vi "MainGUI.vi"() -> ()   [LabVIEW 2018]
uses:
  General/Controls/ScanType.ctl
  General/Controls/Vibratome Parameters.ctl
  General/type defines/vibratome.ctl
  General/Controls/Imaging Parameters.ctl
  General/Controls/Scan Direction.ctl
  General/type defines/Alazar parameters.ctl
  Hardware Mfg/AlazarTech SDK/Controls/General Trigger Settings.ctl
  Hardware Mfg/AlazarTech SDK/Controls/Trigger Engine Controls.ctl
  Hardware Mfg/AlazarTech SDK/Controls/Alazar Device ID.ctl
  Hardware Mfg/AlazarTech SDK/Controls/Channel Input Controls.ctl
  Hardware Mfg/AlazarTech SDK/Controls/Alazar Acquisition Settings.ctl
  Hardware Mfg/AlazarTech SDK/Controls/Clock Controls.ctl
  General/type defines/Galvo HW Parameters.ctl
  General/Controls/Optical Parameters.ctl
  General/Controls/Translation Stage Parameters.ctl
  Hardware Mfg/Thorlabs Translation Stages/Controls/Translation Stage Cluster.ctl
  General/Controls/Translation Stage Types.ctl
  General/type defines/Manual Controls.ctl
  General/type defines/FFT parameters.ctl
  General/type defines/FFT mode.ctl
  General/type defines/GPU FFT outputs.ctl
  General/type defines/Vibratome Param.ctl
  General/type defines/attenuator.ctl
  C:/Project/SerialSectionOCT/SerialSectOCT/Labview Software/Thorlabs.MotionControl.Controls.dll
  Thorlabs.MotionControl.Controls.dll
  General/Controls/Queue Manager Actions.ctl
  General/Controls/MessagePacket.ctl
  General/Controls/QueueNames.ctl
  General/Controls/FGV Actions.ctl
  General/Controls/Save Bline to Mem Control.ctl
  General/Tile naming actions.ctl
  General/type defines/Pause action.ctl
  Hardware Mfg/Thorlabs Cage Rotation/refnum control.ctl
  General/Controls/Set Get Controls.ctl
  Hardware Mfg/Thorlabs Translation Stages/Controls/Motion Translation Module Control2.ctl
  General/Controls/file variable action.ctl
  Hardware Mfg/Main Scan Processor Status.vi
  Hardware Mfg/Axsun Laser/Axsun action.ctl
panel:
  in  "Status":string
  in  "Quit":bool
  in  "Acquire":bool
  in  "Control Panel":T1(tab)
  in  "Optical Parameters":T2={"Obj. Focal Length [mm]"=45.0, "Scan Lens EFL[mm]"=59.5, "Tube Lens EFL[mm]"=205.0, "Galvo V Range (+/-)"=10.0, "Galvo Max Half Angle [Deg]"=19.0, "Max Galvo Range[%]"=0.0}
  in  "Galvo HW Parameters":T3={"Analog Out Channel"="GalvoCtrl/ao0,GalvoCtrl/ao1", "Min Voltage"=-10.0, "Max Voltage"=10.0, "Pixel Clock Source"="/GalvoCtrl/PFI0", "Sample Rate"=1000.0, "Line Clock Out Ch(s)"="GalvoCtrl/port0/line0", "2P ready check"="Dev1/port0/line0:7"}
  in  "Imaging Parameter":T4={"Raster Scan Direction"=enum."Uni Directional", "Pixel Dwell Time [Clock Cycles]"=1, "Flyback Time [Clock Cycles]"=150, "XY Center [um]"={"X"=550.0, "Y"=450.0}, "Pixel Step Size [um] X"=3.0, "XY Image Size"=enum."2048 x 2048", "Custom"=TRUE, "Custom Size"={"X"=1050, "Y"=30}, "Line Averages"=1, "Pixel Step Size [um] Y"=0.0} {"Pixel Step Size [um] Y" min=0.0 max=100.0 step=0.01; "Line Averages" min=1 max=30 step=1; "Flyback Time [Clock Cycles]" max=1000 step=1; "Pixel Step Size [um] X" min=0.0 max=100.0 step=0.01; "Custom Size"."Y" min=2 max=10000 step=1; "Custom Size"."X" min=1 max=30 step=1; "XY Center [um]"."Y" min=1.0 max=30.0 step=1.0; "XY Center [um]"."X" min=1.0 max=30.0 step=1.0; "Pixel Dwell Time [Clock Cycles]" max=10 step=1}
  in  "Scan Type":T6
  in  "Alazar parameters":T7={"Trigger Settings"={"General Trigger Settings"={"Trigger Operation"=0, "Coupling ID"=2, "Range ID"=2, "Delay"=0, "Timeout Ticks"=0, "Mode"=1, "Parameter"=1}, "Trigger Engine 1"={"Trigger Engine"=0, "Source"=2, "Slope"=1, "Level"=140}, "Trigger Engine 2"={"Trigger Engine"=1, "Source"=2, "Slope"=1, "Level"=2048}}, "Device ID"={"System ID"=1, "Board ID"=1}, "Ch A Input Control"={"Channel"=1, "Coupling"=2, "Range"=7, "Impedance"=2}, "Ch B Input Control"={"Channel"=2, "Coupling"=2, "Range"=7, "Impedance"=2}, "Acq Settings"={"Record Length"=1440, "Offset"=0, "Records Per Buffer"=1100, "Records Count (Records/Acq)"=2147483647, "Window Type"=1, "Footer"=0, "Samples per record"=2048, "Output Format"=11}, "Capture Clock"={"Sample Rate"=100, "Decimation"=0, "Source"=2, "Edge"=0}} {"Capture Clock"."Edge" items=["Rising", "Falling"]; "Capture Clock"."Source" items=["Internal"=1, "Fast External"=2, "Medium External"=3, "Slow External"=4, "External AC"=5, "External DC"=6, "External 10MHz"=7]; "Acq Settings"."Output Format" items=["Float Log"=11, "Float Amp"=10, "U16_LOG"=1, "U16_AMP2"=257, "Real"=3, "Imag"=4]; "Acq Settings"."Footer" items=["FOOTER_NONE", "FOOTER_NPT"]; "Acq Settings"."Window Type" items=["DSP_WINDOW_NONE", "DSP_WINDOW_HANNING", "DSP_WINDOW_HAMMING", "DSP_WINDOW_BLACKMAN", "DSP_WINDOW_BLACKMAN_HARRIS", "DSP_WINDOW_BARTLETT"]; "Ch B Input Control"."Channel" items=["A"=1, "B"=2, "C"=4, "D"=8]; "Ch B Input Control"."Coupling" items=["AC"=1, "DC"=2]; "Ch B Input Control"."Range" items=["20 mV"=1, "40 mV"=2, "50 mV"=3, "80 mV"=4, "100 mV"=5, "200 mV"=6, "400 mV"=7, "500 mV"=8, "800 mV"=9, "1 V"=10, "1.25 V"=33, "2 V"=11, "4 V"=12, "5 V"=13, "8 V"=14, "10 V"=15, "20 V"=16]; "Ch B Input Control"."Impedance" items=["1 MOhm"=1, "50 Ohm"=2, ""=0]; "Ch A Input Control"."Channel" items=["A"=1, "B"=2, "C"=4, "D"=8]; "Ch A Input Control"."Coupling" items=["AC"=1, "DC"=2]; "Ch A Input Control"."Range" items=["20 mV"=1, "40 mV"=2, "50 mV"=3, "80 mV"=4, "100 mV"=5, "200 mV"=6, "400 mV"=7, "500 mV"=8, "800 mV"=9, "1 V"=10, "1.25 V"=33, "2 V"=11, "4 V"=12, "5 V"=13, "8 V"=14, "10 V"=15, "20 V"=16]; "Ch A Input Control"."Impedance" items=["1 MOhm"=1, "50 Ohm"=2, ""=0]; "Trigger Settings"."General Trigger Settings"."Trigger Operation" items=["J", "K", "J OR K", "J AND K", "J XOR K", "J AND NOT K", "NOT J AND K"]; "Trigger Settings"."General Trigger Settings"."Coupling ID" items=["AC"=1, "DC"=2]; "Trigger Settings"."General Trigger Settings"."Range ID" items=["5 V", "1 V", "TTL"]; "Trigger Settings"."Trigger Engine 1"."Trigger Engine" items=["J", "K"]; "Trigger Settings"."Trigger Engine 1"."Source" items=["A", "B", "External", "Disable", "C", "D"]; "Trigger Settings"."Trigger Engine 1"."Slope" items=["Positive"=1, "Negative"=2]; "Trigger Settings"."Trigger Engine 2"."Trigger Engine" items=["J", "K"]; "Trigger Settings"."Trigger Engine 2"."Source" items=["A", "B", "External", "Disable", "C", "D"]; "Trigger Settings"."Trigger Engine 2"."Slope" items=["Positive"=1, "Negative"=2]}
  in  "Z stage settings":T14={"first cut height(mm)"=45.85, "slice thickness[um]"=[], "#repetitions"=111, "image thickness(um)"=[], "#cycles per repetition"=0, "First image height(mm)"=2.1, "Block?"=[], "Z0"=0.0, "fixed Z0?"=FALSE}
  in  "Vibratome":T15={"Pre Cut Dwell [s]"=0.0, "Blade Frequency [RPM]"=0, "Slice Speed [mm/s]"=0.0, "Post Cut Dwell [s]"=0.0, "Ramp Time [s]"=10.0, "Start X [mm]"=0.0, "Start Y [mm]"=0.0, "Slice Length [mm]"=0.0, "Slice Axis"=enum."X Axis", "Controller VISA Ref"="COM4", "Blade Frequency [Hz]"=0, "Analog Out Channel"="GalvoCtrl/ao0,GalvoCtrl/ao1", "Pixel Clock Source"="/GalvoCtrl/PFI0", "Vib version"=enum."Vibratome1"} {"Start X [mm]" min=10.0; "Slice Speed [mm/s]" format="%.2f"}
  in  "Mosaic Paramter":T17={"X Axis"={"Start [mm]"=56.0, "FOV[mm]"=3.0, "End [mm]"=70.8}, "Y Axis"={"Start [mm]"=102.5, "FOV[mm]"=3.0, "End [mm]"=117.2}, "Scan Pattern"=enum."Uni-directional", "Overlap Options"={"Overlap Type"=enum."X and Y", "Percent Overlap"=10, "Justify"=enum."Start"}}
  in  "Attenuator":T18
  in  "Manual Controls":T19={"Data Path"=path "C:/Users/BOAS-USER/Documents/Data/0922", "Save parameters"={"start pixel"=45, "#pixels to save"=100}, "Acquisition mode"=enum."Alazar FFT", "PSOCT Channel"=1, "Save data?"=FALSE, "AIP rotation angle"=0.0, "Pause acquisition?"=FALSE, "Outgoing Mail Server (SMTP)"="smtp.gmail.com", "Email"="nauge7811@gmail.com", "Password"="csb19960128", "Carrier 1"=enum."Sprint", "phone number 1"="8578002084", "Subject"="", "Message"="Brain slice: stop watching Netflix, come and pick me up!", "Carrier 2"=enum."Sprint", "phone number 2"="", "Check boundary?"=FALSE, "Threshold"=0.0, "Outputs for GPU FFT"=enum."Amp + Phase diff"} {"PSOCT Channel" items=["A"=1, "B"=2, "A + B"=3, "C"=4, "A + C"=5, "A + B"=6, "D"=8, "A + D"=9, "B + D"=10, "C + D"=12, "A + B + C + D"=15]}
  in  "Table Stages":T23={"X Stage"={"Position"=0.0, "Is.Enabled?"=FALSE, "Is.Connected?"=FALSE, "Device SN"="45876425", "AccelerationMaximum"=20.0, "VelocityMaximum"=20.0, "Acceleration"=10.0, "Velocity"=10.0, "waitTimeout (ms)"=1000000, "Model"=enum."Thorlabs LTS", "Is.Homed?"=FALSE, "MOVE"=FALSE}, "Y Stage"={"Position"=0.0, "Is.Enabled?"=FALSE, "Is.Connected?"=FALSE, "Device SN"="45995820", "AccelerationMaximum"=20.0, "VelocityMaximum"=20.0, "Acceleration"=10.0, "Velocity"=10.0, "waitTimeout (ms)"=10000000, "Model"=enum."Thorlabs LTS", "Is.Homed?"=FALSE, "MOVE"=FALSE}, "Z Stage"={"Position"=0.0, "Is.Enabled?"=FALSE, "Is.Connected?"=FALSE, "Device SN"="49103464", "AccelerationMaximum"=8.0, "VelocityMaximum"=3.0, "Acceleration"=4.0, "Velocity"=2.0, "waitTimeout (ms)"=1000000, "Model"=enum."Thorlabs MLJ", "Is.Homed?"=FALSE, "MOVE"=FALSE}, "Attenuator"={"Position"=0.0, "Is.Enabled?"=FALSE, "Is.Connected?"=FALSE, "Device SN"="45876539", "AccelerationMaximum"=0.0, "VelocityMaximum"=0.0, "Acceleration"=0.0, "Velocity"=0.0, "waitTimeout (ms)"=0, "Model"=enum."None", "Is.Homed?"=FALSE, "MOVE"=FALSE}}
  in  "Attenuator":refnum<k24>(container)
  out "XY Graph out":cluster{"X":dbl, "Y":dbl}[](graph)
  out "AIP":T26(plugin-control) caption="Image"
  out "wanring":string="test"
  out "attenuator angle":dbl
  in  "attenuator power(mW)":dbl=300.0 format="%#_13g"
  out "requested 2P power out":dbl
  out "attenuator angle out":dbl
  out "tile average intensity":dbl
  in  "Init Tables":bool
  out "Current Position out":cluster{"X":dbl, "Y":dbl, "Z":dbl}
  out "slice plane out":dbl
  out "image plane out":dbl
  # "Image Settings"
  # "Optical Settings"
  # "X"
  # "X"
  # "(mW)"
  # "Vibratome Settings"
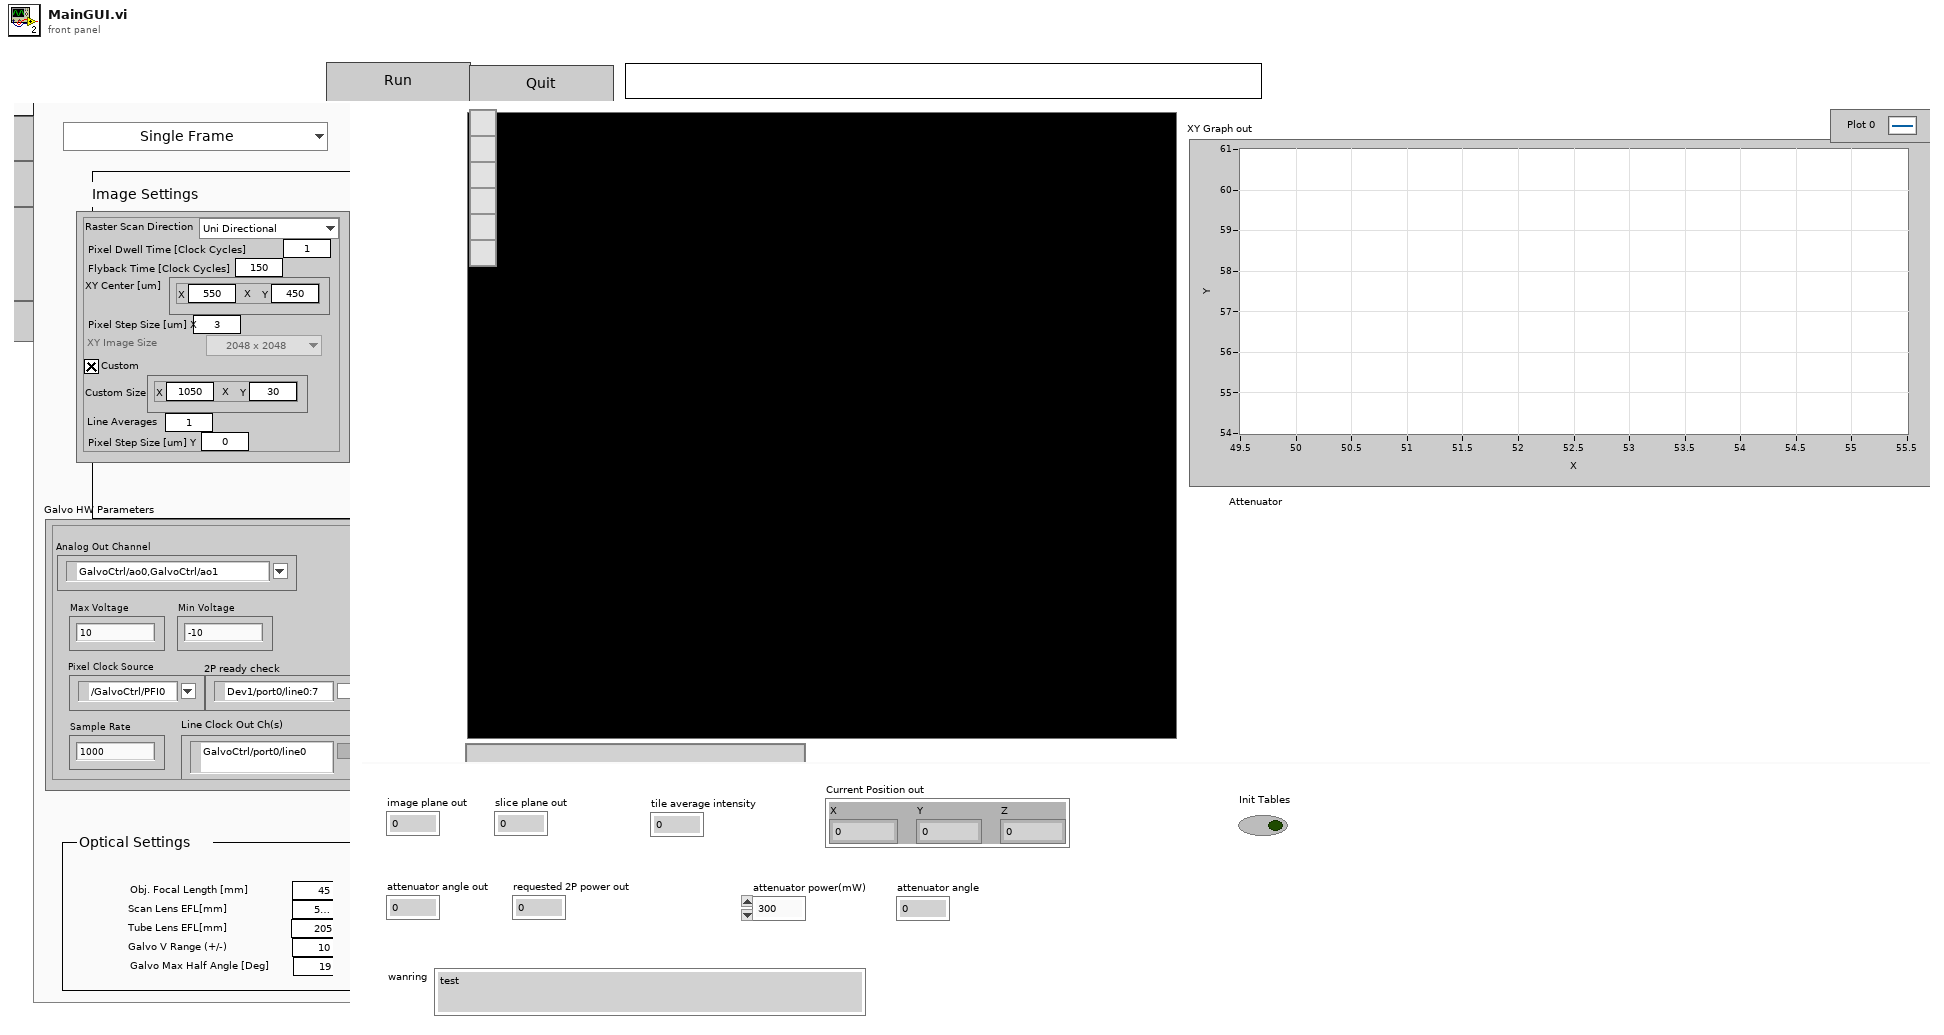
[diagram p1: front panel]
types:
  T1 = enum32{"Galvo", "Alazar", "Config", "Manual Contorls", "Table"}
  T2 = typedef "Optical Parameters.ctl" = cluster{"Obj. Focal Length [mm]":dbl, "Scan Lens EFL[mm]":dbl, "Tube Lens EFL[mm]":dbl, "Galvo V Range (+/-)":dbl, "Galvo Max Half Angle [Deg]":dbl, "Max Galvo Range[%]":dbl}
  T3 = typedef "Galvo HW Parameters.ctl" = cluster{"Analog Out Channel":tag, "Min Voltage":dbl, "Max Voltage":dbl, "Pixel Clock Source":tag, "Sample Rate":dbl, "Line Clock Out Ch(s)":tag, "2P ready check":tag}
  T4 = typedef "Imaging Parameters.ctl" = cluster{"Raster Scan Direction":T5, "Pixel Dwell Time [Clock Cycles]":u16, "Flyback Time [Clock Cycles]":u16, "XY Center [um]":cluster{"X":dbl, "Y":dbl}, "Pixel Step Size [um] X":dbl, "XY Image Size":enum16{"32 x 32", "64 x 64", "128 x 128", "256 x 256", "512 x 512", "1024 x 1024", "2048 x 2048"}, "Custom":bool, "Custom Size":cluster{"X":u16, "Y":u16}, "Line Averages":u16, "Pixel Step Size [um] Y":dbl}
  T5 = typedef "Scan Direction.ctl" = enum16{"Uni Directional", "Bi Directional", "None"}
  T6 = typedef "ScanType.ctl" = enum16{"Single Frame", "Continuous Frame", "ROI Line", "Vibratome", "Mosaic", "Mosaic + Slice"}
  T7 = typedef "Alazar parameters.ctl" = cluster{"Trigger Settings":cluster{"General Trigger Settings":T8, "Trigger Engine 1":T9, "Trigger Engine 2":T9}, "Device ID":T10, "Ch A Input Control":T11, "Ch B Input Control":T11, "Acq Settings":T12, "Capture Clock":T13}
  T8 = typedef "General Trigger Settings.ctl" = cluster{"Trigger Operation":u32, "Coupling ID":u32, "Range ID":u32, "Delay":u32, "Timeout Ticks":u32, "Mode":u32, "Parameter":u32}
  T9 = typedef "Trigger Engine Controls.ctl" = cluster{"Trigger Engine":u32, "Source":u32, "Slope":u32, "Level":u32}
  T10 = typedef "Alazar Device ID.ctl" = cluster{"System ID":u32, "Board ID":u32}
  T11 = typedef "Channel Input Controls.ctl" = cluster{"Channel":u8, "Coupling":u32, "Range":u32, "Impedance":u32}
  T12 = typedef "Alazar Acquisition Settings.ctl" = cluster{"Record Length":u32, "Offset":u32, "Records Per Buffer":u32, "Records Count (Records/Acq)":u32, "Window Type":u32, "Footer":u32, "Samples per record":u32, "Output Format":u32}
  T13 = typedef "Clock Controls.ctl" = cluster{"Sample Rate":u32, "Decimation":u32, "Source":u32, "Edge":u32}
  T14 = typedef "Vibratome Param.ctl" = cluster{"first cut height(mm)":dbl, "slice thickness[um]":dbl[], "#repetitions":u16, "image thickness(um)":dbl[], "#cycles per repetition":u16, "First image height(mm)":dbl, "Block?":bool[], "Z0":dbl, "fixed Z0?":bool}
  T15 = typedef "Vibratome Parameters.ctl" = cluster{"Pre Cut Dwell [s]":dbl, "Blade Frequency [RPM]":u16, "Slice Speed [mm/s]":dbl, "Post Cut Dwell [s]":dbl, "Ramp Time [s]":dbl, "Start X [mm]":dbl, "Start Y [mm]":dbl, "Slice Length [mm]":dbl, "Slice Axis":enum16{"X Axis", "Y Axis", "Z Axis"}, "Controller VISA Ref":refnum<visa-resource-name>, "Blade Frequency [Hz]":u16, "Analog Out Channel":tag, "Pixel Clock Source":tag, "Vib version":T16}
  T16 = typedef "vibratome.ctl" = enum16{"Vibratome1", "Vibratome3"}
  T17 = cluster{"X Axis":cluster{"Start [mm]":dbl, "FOV[mm]":dbl, "End [mm]":dbl}, "Y Axis":cluster{"Start [mm]":dbl, "FOV[mm]":dbl, "End [mm]":dbl}, "Scan Pattern":enum16{"Uni-directional", "Bi-Directional", "Spiral Out", "Spiral In"}, "Overlap Options":cluster{"Overlap Type":enum16{"No Overlap", "X Only", "Y Only", "X and Y"}, "Percent Overlap":u8, "Justify":enum16{"Start", "Center", "End"}}}
  T18 = typedef "attenuator.ctl" = cluster{"Power after Objective (recalibrate every 6 month)":dbl[]}
  T19 = typedef "Manual Controls.ctl" = cluster{"Data Path":path, "Save parameters":T20, "Acquisition mode":T21, "PSOCT Channel":u32, "Save data?":bool, "AIP rotation angle":dbl, "Pause acquisition?":bool, "Outgoing Mail Server (SMTP)":string, "Email":string, "Password":string, "Carrier 1":enum16{"T-Mobile", "AT&T", "Verizon", "Sprint"}, "phone number 1":string, "Subject":string, "Message":string, "Carrier 2":enum16{"T-Mobile", "AT&T", "Verizon", "Sprint"}, "phone number 2":string, "Check boundary?":bool, "Threshold":sgl, "Outputs for GPU FFT":T22}
  T20 = typedef "FFT parameters.ctl" = cluster{"start pixel":i32, "#pixels to save":i32}
  T21 = typedef "FFT mode.ctl" = enum16{"ThorOCT B line", "ThorOCT Spectral", "ThorOCT FFT", "Alazar B line", "Alazar FFT", "GPU FFT", "Alazar Spectral", "Simulation", "auto adjust focus", "Save all"}
  T22 = typedef "GPU FFT outputs.ctl" = enum16{"Amp + Phase diff", "Amp + Phase", "Amp only"}
  T23 = typedef "Translation Stage Parameters.ctl" = cluster{"X Stage":T24, "Y Stage":T24, "Z Stage":T24, "Attenuator":T24}
  T24 = typedef "Translation Stage Cluster.ctl" = cluster{"Position":dbl, "Is.Enabled?":bool, "Is.Connected?":bool, "Device SN":string, "AccelerationMaximum":dbl, "VelocityMaximum":dbl, "Acceleration":dbl, "Velocity":dbl, "waitTimeout (ms)":i32, "Model":T25, "Is.Homed?":bool, "MOVE":bool}
  T25 = typedef "Translation Stage Types.ctl" = enum16{"None", "Thorlabs LTS", "Thorlabs MLJ"}
  T26 = typedef "IMAQ Image.ctl" = refnum<image>
  T27 = enum16{"Create file", "Write config", "Write log", "Close file"}
  T28 = typedef "Queue Manager Actions.ctl" = enum16{"Init", "Enqueue", "Enqueue All", "Preview Queue", "Dequeue", "Get Status", "Flush Queue", "Flush All Queues", "Release All Queues", "Release Queue", "Enqueue at Opposite End"}
  T29 = typedef "QueueNames.ctl" = enum16{"Main GUI", "Main Scan Processor", "Main Processing", "Main Saving", "Main Display", "Main Table Stage GUI", "Main Table Stage Proc.", "Scan Engine", "Vibratome GUI", "Vibratome Processor", "Slice Engine"}
  T30 = typedef "MessagePacket.ctl" = cluster{"Message":string, "Parameter":variant}
  T31 = typedef "FGV Actions.ctl" = enum16{"Init", "Set", "Get", "Clear"}
  T32 = typedef "Image Type" = u32
  T33 = typedef "System Parameters.ctl" = cluster{"Optical Parameters":T2, "Vibratome":T15, "Table Stages":T23, "Imaging Parameter":T4, "Galvo HW Parameters":cluster{"Analog Out Channel":tag, "Min Voltage":dbl, "Max Voltage":dbl, "Pixel Clock Source":tag, "Sample Rate":dbl, "Line Clock Out Ch":tag, "2P ready check":tag}, "Alazar parameters":T7, "Mosaic Paramter":cluster{"X Axis":cluster{"Start [mm]":dbl, "Steps [pts]":dbl, "End [mm]":dbl}, "Y Axis":cluster{"Start [mm]":dbl, "Steps [pts]":dbl, "End [mm]":dbl}, "Scan Pattern":enum16{"Uni-directional", "Bi-Directional", "Spiral Out", "Spiral In"}, "Overlap Options":cluster{"Overlap Type":enum16{"No Overlap", "X Only", "Y Only", "X and Y"}, "Percent Overlap":u8, "Justify":enum16{"Start", "Center", "End"}}}, "Manual Controls":T19, "Z stage setting":T14, "Attenuator":T18}
  T34 = typedef "file variable action.ctl" = enum16{"File name", "X stage", "Y stage", "Slice plane", "Image plane", "time", "output", "Init", "Memory Usage", "Disk full Space", "Disk free space"}
  T35 = typedef "Pause action.ctl" = enum16{"Init", "get", "set"}
  T36 = typedef "Tile naming actions.ctl" = enum16{"Export", "Increment", "Total tile num", "Init"}
  T37 = typedef "Axsun action.ctl" = enum16{"GetSystemStatus", "Clock delay", "GetLaserOnTime", "GetWaveLengthAtSweptTrigger", "Source current ON", "GetSerialNum", "GetControlVersion", "Laser ON", "Laser OFF", "Source current OFF", "Get laser handle", "Start Network Control Interface", "stop", "Create handle"}
  T38 = typedef "Save Bline to Mem Control.ctl" = enum16{"Output data", "Save(ThorOCT)", "Save(PSOCT)", "FFT and Save", "Uninit", "PSOCT Spectral buffer Set", "PSOCT Spatial buffer Set", "PSOCT Spectral buffer Init", "PSOCT Spatial buffer Init", "ThorOCT Spectral buffer Init", "ThorOCT Spatial buffer Init", "ThorOCT Spectral buffer Set", "ThorOCT Spatial buffer Set", "ThorOCT Spectral Save", "Alazar Spectral Save", "PSOCT save all", "Average"}
  T39 = typedef "refnum control.ctl" = enum16{"Get", "Init"}
  T40 = typedef "Motion Translation Module Control2.ctl" = enum16{"Init", "Home", "Status", "Velocity/Accel", "Position", "Jog", "Stop", "Uninit", "Enable", "Disable"}
  T41 = typedef "Set Get Controls.ctl" = enum16{"Set", "Get"}
  T42 = cluster{"Analog Out Channel":tag, "Min Voltage":dbl, "Max Voltage":dbl, "Pixel Clock Source":tag, "Sample Rate":dbl, "Line Clock Out Ch":tag, "2P ready check":tag}
  T43 = cluster{"X Axis":cluster{"Start [mm]":dbl, "Steps [pts]":dbl, "End [mm]":dbl}, "Y Axis":cluster{"Start [mm]":dbl, "Steps [pts]":dbl, "End [mm]":dbl}, "Scan Pattern":enum16{"Uni-directional", "Bi-Directional", "Spiral Out", "Spiral In"}, "Overlap Options":cluster{"Overlap Type":enum16{"No Overlap", "X Only", "Y Only", "X and Y"}, "Percent Overlap":u8, "Justify":enum16{"Start", "Center", "End"}}}
  T44 = enum16{"32 x 32", "64 x 64", "128 x 128", "256 x 256", "512 x 512", "1024 x 1024", "2048 x 2048"}
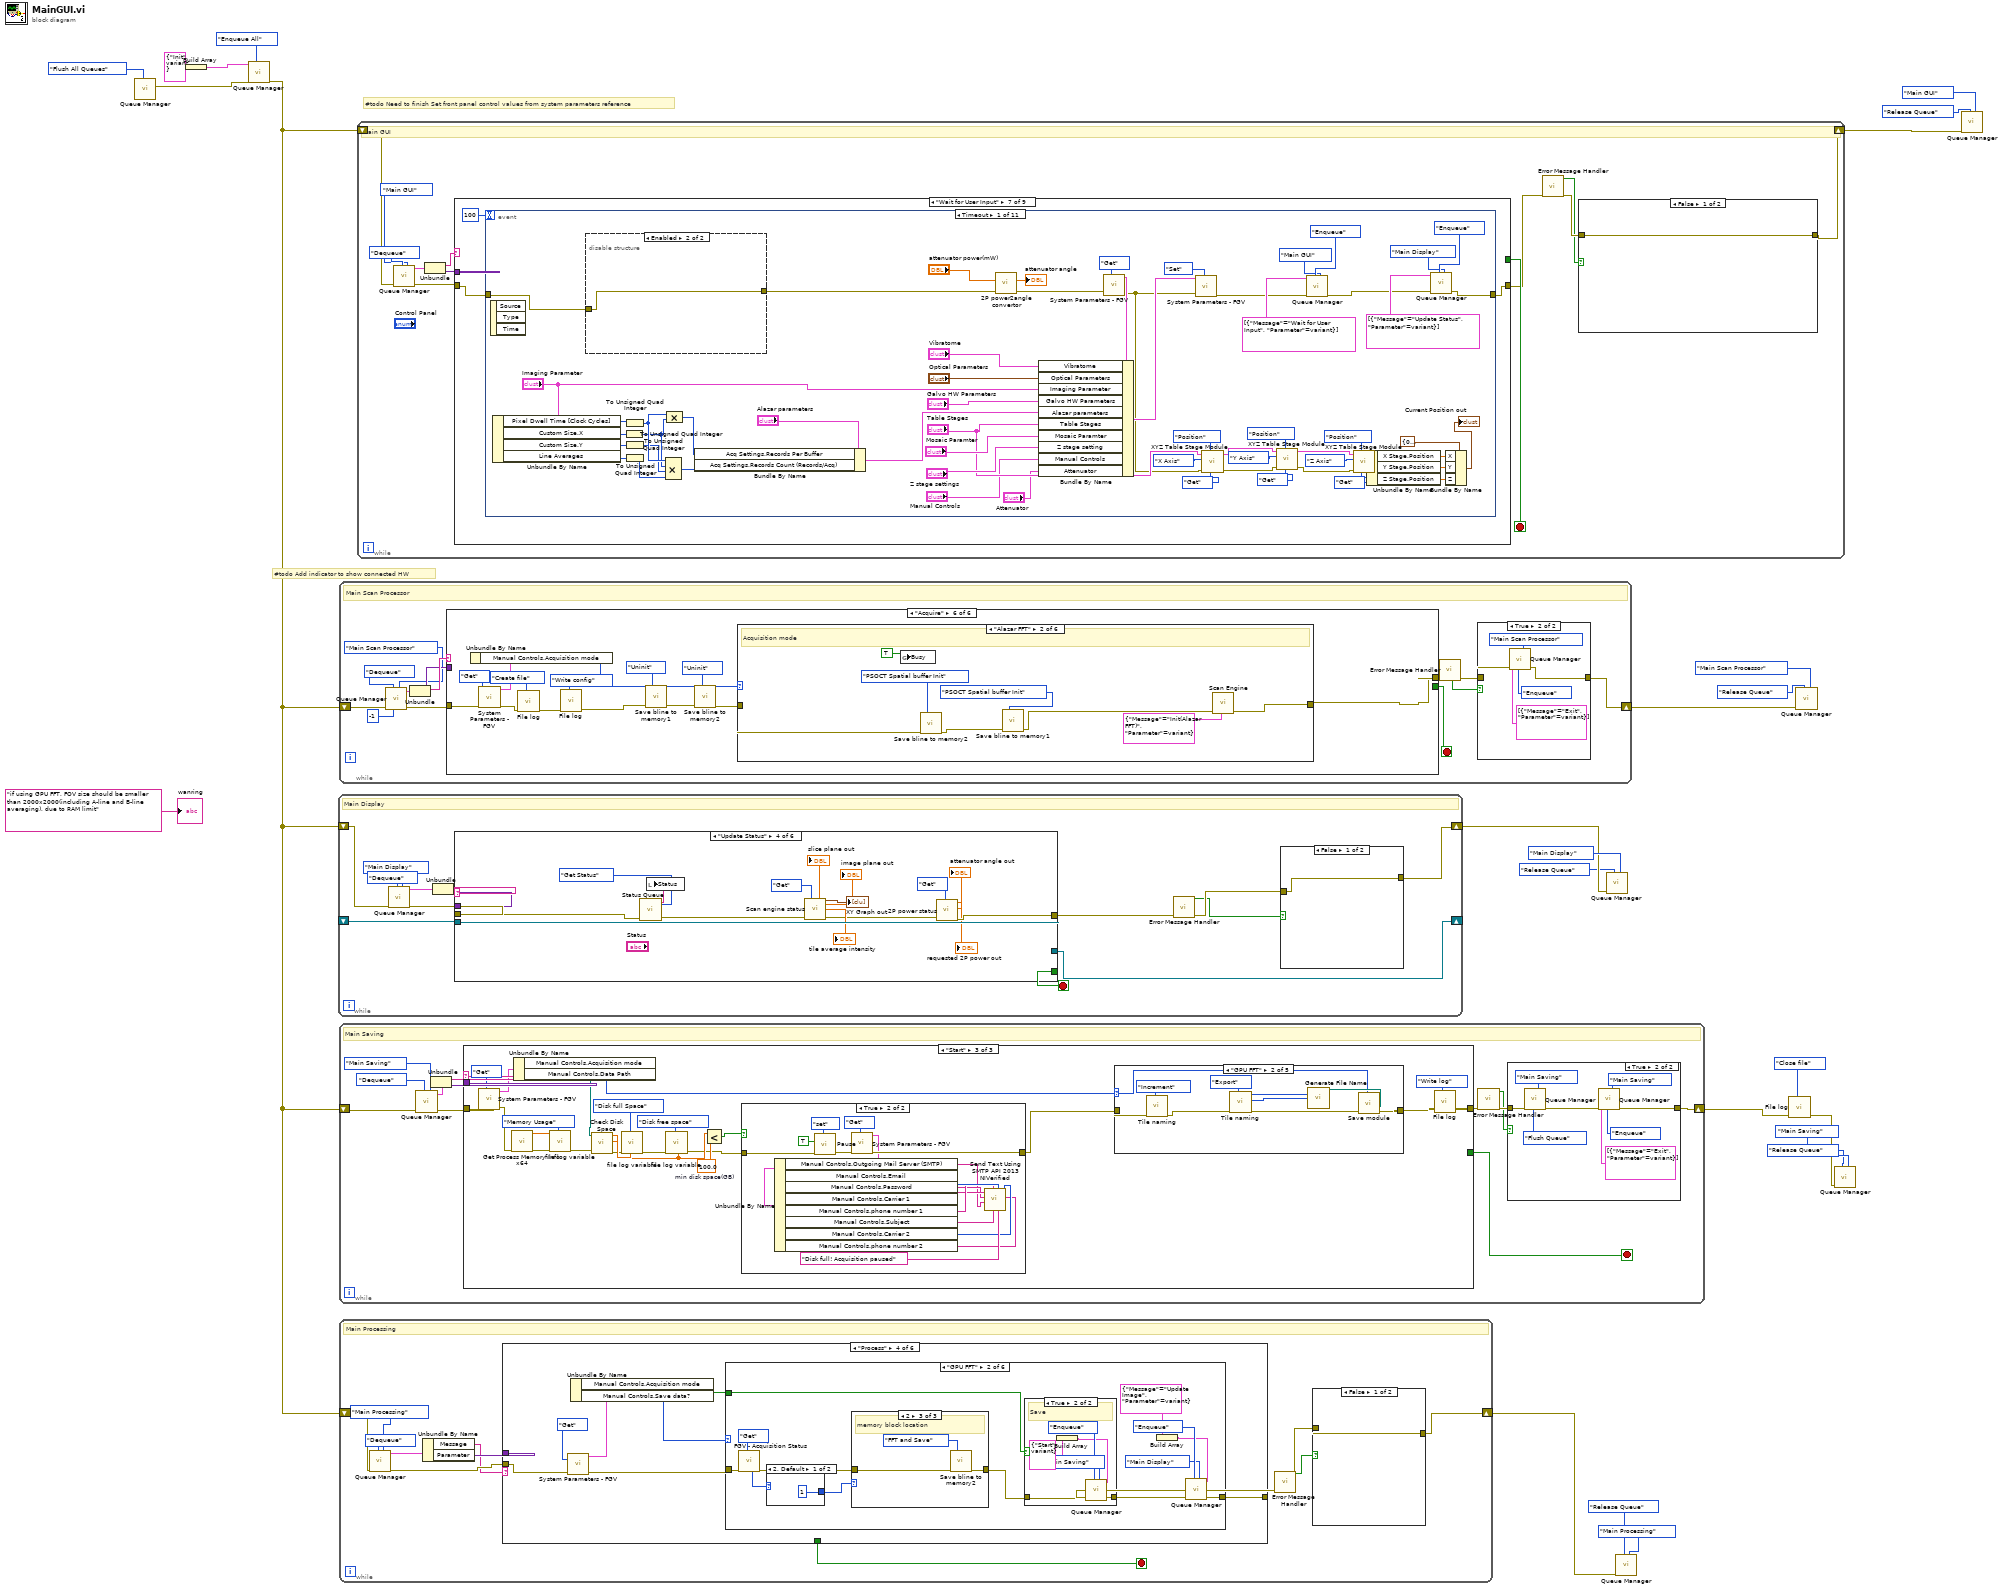
[diagram p0: block diagram]
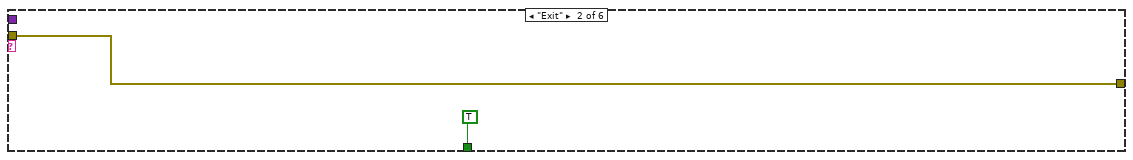
[diagram p3: hidden frame]
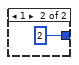
[diagram p6: hidden frame]
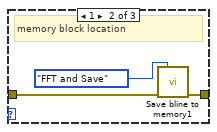
[diagram p9: hidden frame]
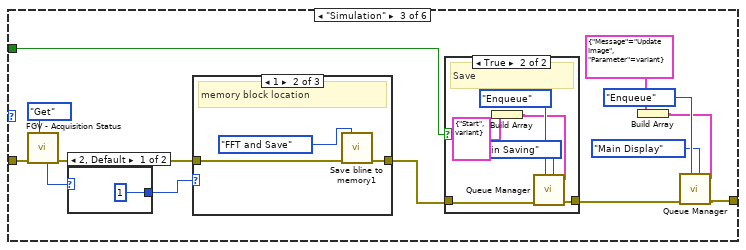
[diagram p10: hidden frame]
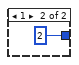
[diagram p11: hidden frame]
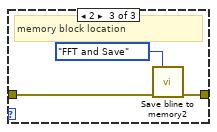
[diagram p14: hidden frame]
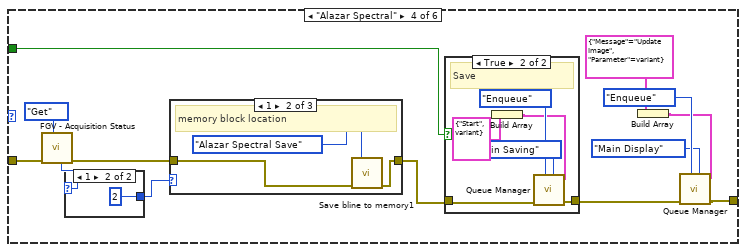
[diagram p15: hidden frame]
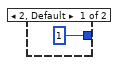
[diagram p16: hidden frame]
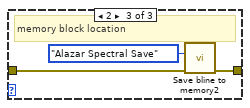
[diagram p19: hidden frame]
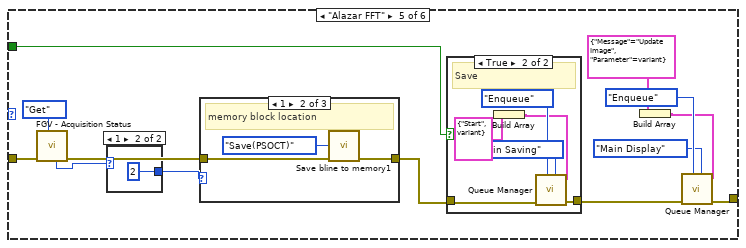
[diagram p20: hidden frame]
diagram:
  # "#todo Add indicator to show connected HW"
  # "#todo Need to finish Set front panel control values from system parameters reference"
  n1 = call "Queue Manager.vi"("Action"=Queue_Manager_Actions."Flush All Queues") -> ("Error Out"=w6:errorcluster)  [unwired: 6 in, 4 out]
  n2 = Build Array(T30 {"Message"="Init", "Parameter"=variant} ("Message Packet [In]")) -> (w22:T30[])
  n3 = call "Queue Manager.vi"("Action"=Queue_Manager_Actions."Enqueue All", "Error In"=w6, "Message Packet Array"=w22) -> ("Error Out"=w2:errorcluster)  [unwired: 4 in, 4 out]
  n4 = while {
    shift-right: [w27] -> w14
    shift-left: w2 -> [w35]
    shift-right: [w37] -> _
    shift-left: _ -> [w36]
    stop <- w38 stop-if-true
    # "Main Display"
    n5 = call "Queue Manager.vi"("Queue Name"=QueueNames."Main Display", "Action"=Queue_Manager_Actions."Dequeue", "Error In"=w35) -> ("Error Out"=w32:errorcluster, "Message Packet [Out]"=w31:T30)  [unwired: 4 in, 3 out]
    n6 = Unbundle(w31) -> ("Message"=w30:string, "Parameter"=w29:variant)
    n7 = case shown="\"Update Status\"" w30 {
      tunnel: w32 -> [w49 w52 w63 w105 w107 w109]
      tunnel: w29 -> [_ _ _ _ _ _]
      tunnel: [w47 w53 w66 w94 w107 w109] -> w25
      tunnel: [TRUE _ _ _ _ _] -> w38
      tunnel: [_ w55 w68 w102 w106 w108] -> w37
      tunnel: w36 -> [_ _ w68 w102 w106 w108]
      frame "Exit" {
        n8 = call "RAW Image Buffer.vi"("Actions"=enum16{"Init", "Create", "Get", "Dispose"}."Dispose", "Error In"=w49) -> ("Error Out"=w48:errorcluster, "Image Out"=w45:T26)  [unwired: 8 in]
        n9 = local write "AIP"(w45) -> ()
        n10 = call "Image Queue.vi"("Action"=Queue_Manager_Actions."Release Queue", "Error In"=w48) -> ("Error Out"=w47:errorcluster)  [unwired: 8 in, 1 out]
      }
      frame "Init" {
        w56 = T32 2 items=["Grayscale (U8)", "Grayscale (I16)", "Grayscale (SGL)", "Complex (CSG)", "RGB (U32)", "HSL (U32)", "RGB (U64)", "Grayscale (U16)"] ("Image Type")
        n11 = call "RAW Image Buffer.vi"("Actions"=enum16{"Init", "Create", "Get", "Dispose"}."Init", "Error In"=w52) -> ("Error Out"=w60:errorcluster)  [unwired: 8 in, 1 out]
        n12 = call "RAW Image Buffer.vi"("Actions"=enum16{"Init", "Create", "Get", "Dispose"}."Create", "Error In"=w60) -> ("Error Out"=w54:errorcluster)  [unwired: 8 in, 1 out]
        n13 = call "IMAQ Create"("Image Name"="test", "Image Type"=w56, "error in (no error)"=w54) -> ("New Image"=w55:T26, "error out"=w53:errorcluster)  [unwired: 2 in]
      }
      frame "Update Image" {
        n14 = call "System Parameters - FGV.vi"("Actions"=FGV_Actions."Get", "Error In"=w63) -> ("Error Out"=w65:errorcluster, "System Parameters [Out]"=w62:T33)  [unwired: 8 in]
        n15 = Unbundle By Name(w62) -> ("Manual Controls.Acquisition mode"=w61:T21)
        n16 = case shown="\"Alazar FFT\", Default" w61 {
          tunnel: w68 -> [w72 w73 w77 w81 w88 w90]
          tunnel: [w71 w76 w80 w84 w87 w90] -> w67
          tunnel: [w70 w75 w79 w83 w86 w89] -> w66
          tunnel: w65 -> [w69 w74 w78 w82 w85 w89]
          frame "Alazar FFT", Default {
            n17 = call "Display_Module.vi"("error in"=w69, "Source in"=w72) -> ("error out"=w70:errorcluster, "AIP"=w71:T26)  [unwired: 8 in]
          }
          frame "GPU FFT" {
            n18 = call "Display_Module.vi"("error in"=w74, "Source in"=w73) -> ("error out"=w75:errorcluster, "AIP"=w76:T26)  [unwired: 8 in]
          }
          frame "Save all" {
            n19 = call "Display_Module.vi"("error in"=w78, "Source in"=w77) -> ("error out"=w79:errorcluster, "AIP"=w80:T26)  [unwired: 8 in]
          }
          frame "Simulation" {
            n20 = call "Display_Module.vi"("error in"=w82, "Source in"=w81) -> ("error out"=w83:errorcluster, "AIP"=w84:T26)  [unwired: 8 in]
          }
          frame "Alazar B line" {
            n21 = call "Display_Module.vi"("error in"=w85, "Source in"=w88) -> ("error out"=w86:errorcluster, "AIP"=w87:T26)  [unwired: 8 in]
          }
          frame "Alazar Spectral" {
          }
        }
        "AIP" <- w67
      }
      frame "Update Status" {
        n22 = call "Status Queue.vi"("Action"=Queue_Manager_Actions."Get Status", "Error In"=w105) -> ("Error Out"=w99:errorcluster, "Status Message [Out]"=w103:string)  [unwired: 8 in]
        n23 = local write "Status"(w103) -> ()
        n24 = call "Scan engine status.vi"("Actions"=FGV_Actions."Get", "Error In"=w99) -> ("slice plane out"=→"slice plane out":dbl, "image plane out"=→"image plane out":dbl, "XY Graph out"=→"XY Graph out":cluster{"X":dbl, "Y":dbl}[], "average out"=→"tile average intensity":dbl, "Error Out"=w95:errorcluster)  [unwired: 7 in, 2 out]
        n25 = call "2P power status.vi"("Actions"=FGV_Actions."Get", "Error In"=w95) -> ("Error Out"=w94:errorcluster, "attenuator angle out"=→"attenuator angle out":dbl, "requested 2P power out"=→"requested 2P power out":dbl)  [unwired: 7 in]
      }
      frame "Update Line Profile" {
      }
      frame "Idle", Default {
      }
    }
    n26 = call "Error Message Handler.vi"("Error In"=w25) -> ("Error Out"=w28:errorcluster, "T button?"=w26:bool)  [unwired: 9 in]
    n27 = case shown="False" w26 {
      tunnel: [w39 w42] -> w27
      tunnel: w28 -> [w39 w40]
      frame False {
      }
      frame True {
        n28 = call "Queue Manager.vi"("Queue Name"=QueueNames."Main Display", "Action"=Queue_Manager_Actions."Enqueue", "Error In"=w40, "Message Packet Array"=T30[] [{"Message"="Exit", "Parameter"=variant}] ("Message Packet [In]")) -> ("Error Out"=w42:errorcluster)  [unwired: 3 in, 4 out]
      }
    }
  }
  n29 = while {
    shift-right: [w113] -> w4
    shift-left: w2 -> [w110]
    stop <- w111 stop-if-true
    # "Main Saving"
    n30 = call "Queue Manager.vi"("Queue Name"=QueueNames."Main Saving", "Action"=Queue_Manager_Actions."Dequeue", "Error In"=w110) -> ("Error Out"=w117:errorcluster, "Message Packet [Out]"=w121:T30)  [unwired: 4 in, 3 out]
    n31 = Unbundle(w121) -> ("Message"=w112:string, "Parameter"=w118:variant)
    n32 = case shown="\"Start\"" w112 {
      tunnel: [w131 _ w138] -> w114
      tunnel: w118 -> [_ _ _]
      tunnel: w117 -> [w131 _ w154]
      tunnel: [_ TRUE _] -> w111
      frame "False", Default {
      }
      frame "Exit" {
      }
      frame "Start" {
        w136 = 100.0  # min disk space(GB)
        n33 = call "System Parameters - FGV.vi"("Actions"=FGV_Actions."Get", "Error In"=w154) -> ("Error Out"=w146:errorcluster, "System Parameters [Out]"=w153:T33)  [unwired: 8 in]
        n34 = call "Get Process Memory Info x64.vi"("error in (no error)"=w146) -> ("error out"=w145:errorcluster, "Memory Usage by Labview(GB)"=w148:dbl)  [unwired: 8 in, 1 out]
        n35 = Unbundle By Name(w153) -> ("Manual Controls.Acquisition mode"=w152:T21, "Manual Controls.Data Path"=w141:path)
        n36 = call "file log variable.vi"("memory usage"=w148, "error in"=w145, "Item"=file_variable_action."Memory Usage") -> ("error out"=w144:errorcluster)  [unwired: 15 in, 1 out]
        n37 = call "Check Disk Space.vi"("error in"=w144, "path"=w141) -> ("error out"=w143:errorcluster, "Free space"=w137:dbl, "Full Disk Space"=w147:dbl)  [unwired: 7 in]
        n38 = call "file log variable.vi"("error in"=w143, "Item"=file_variable_action."Disk full Space", "Disk full space"=w147) -> ("error out"=w142:errorcluster)  [unwired: 15 in, 1 out]
        n39 = call "file log variable.vi"("error in"=w142, "Item"=file_variable_action."Disk free space", "Disk free space"=w137) -> ("error out"=w135:errorcluster)  [unwired: 15 in, 1 out]
        n40 = Less?(x=w137, y=w136) -> (x < y?=w134:bool)
        n41 = case shown="True" w134 {
          tunnel: w135 -> [w156 w170]
          tunnel: [w156 w168] -> w133
          frame False {
          }
          frame True {
            n42 = call "Pause.vi"("action"=Pause_action."set", "error in"=w170, "Pause!"=TRUE) -> ("error out"=w169:errorcluster)  [unwired: 7 in, 1 out]
            n43 = call "System Parameters - FGV.vi"("Actions"=FGV_Actions."Get", "Error In"=w169) -> ("Error Out"=w168:errorcluster, "System Parameters [Out]"=w166:T33)  [unwired: 8 in]
            n44 = Unbundle By Name(w166) -> ("Manual Controls.Outgoing Mail Server (SMTP)"=w160:string, "Manual Controls.Email"=w163:string, "Manual Controls.Password"=w162:string, "Manual Controls.Carrier 1"=w165:enum16{"T-Mobile", "AT&T", "Verizon", "Sprint"}, "Manual Controls.phone number 1"=w164:string, "Manual Controls.Subject"=w161:string, "Manual Controls.Carrier 2"=w158:enum16{"T-Mobile", "AT&T", "Verizon", "Sprint"}, "Manual Controls.phone number 2"=w157:string)
            n45 = call "Send Text Using SMTP API 2013 NIVerified.vi"("phone number 2"=w157, "Carrier 2"=w158, "Body"="Disk full! Acquisition paused", "Carrier 1"=w165, "Subject"=w161, "phone number 1"=w164, "Outgoing Mail Server (SMTP)"=w160, "Password"=w162, "Email"=w163) -> ()  [unwired: 3 in]
          }
        }
        n46 = case shown="\"GPU FFT\"" w152 {
          selector: w152 -> [w176 w183 w193 _ w218]
          tunnel: [w182 w192 w202 w209 w224] -> w139
          tunnel: w133 -> [w174 w185 w195 w204 w216]
          frame "Alazar FFT", Default {
            n47 = call "Tile naming.vi"(7:Tile_naming_actions."Increment", "Error In"=w174) -> ("Error Out"=w173:errorcluster)  [unwired: 6 in, 3 out]
            n48 = call "Tile naming.vi"(7:Tile_naming_actions."Export", "Error In"=w173) -> ("Error Out"=w177:errorcluster, "tile"=w178:i32, "slice"=w179:i32)  [unwired: 6 in, 1 out]
            n49 = call "Generate File Name.vi"("slice"=w179, "tile"=w178) -> ("appended path"=w181:path)  [unwired: 13 in]
            n50 = call "Save module.vi"("Acquisition mode"=w176, "error in"=w177, "path"=w181) -> ("error out"=w182:errorcluster)  [unwired: 8 in]
          }
          frame "GPU FFT" {
            n51 = call "Tile naming.vi"(7:Tile_naming_actions."Increment", "Error In"=w185) -> ("Error Out"=w184:errorcluster)  [unwired: 6 in, 3 out]
            n52 = call "Tile naming.vi"(7:Tile_naming_actions."Export", "Error In"=w184) -> ("Error Out"=w187:errorcluster, "tile"=w188:i32, "slice"=w189:i32)  [unwired: 6 in, 1 out]
            n53 = call "Generate File Name.vi"("slice"=w189, "tile"=w188) -> ("appended path"=w191:path)  [unwired: 13 in]
            n54 = call "Save module.vi"("Acquisition mode"=w183, "error in"=w187, "path"=w191) -> ("error out"=w192:errorcluster)  [unwired: 8 in]
          }
          frame "Simulation" {
            n55 = call "Tile naming.vi"(7:Tile_naming_actions."Increment", "Error In"=w195) -> ("Error Out"=w194:errorcluster)  [unwired: 6 in, 3 out]
            n56 = call "Tile naming.vi"(7:Tile_naming_actions."Export", "Error In"=w194) -> ("Error Out"=w197:errorcluster, "tile"=w198:i32, "slice"=w199:i32)  [unwired: 6 in, 1 out]
            n57 = call "Generate File Name.vi"("slice"=w199, "tile"=w198) -> ("appended path"=w201:path)  [unwired: 13 in]
            n58 = call "Save module.vi"("Acquisition mode"=w193, "error in"=w197, "path"=w201) -> ("error out"=w202:errorcluster)  [unwired: 8 in]
          }
          frame "Alazar Spectral" {
            n59 = call "Tile naming.vi"(7:Tile_naming_actions."Increment", "Error In"=w204) -> ("Error Out"=w203:errorcluster)  [unwired: 6 in, 3 out]
            n60 = call "Tile naming.vi"(7:Tile_naming_actions."Export", "Error In"=w203) -> ("Error Out"=w210:errorcluster, "tile"=w211:i32, "slice"=w212:i32)  [unwired: 6 in, 1 out]
            n61 = call "Generate File Name.vi"("slice"=w212, "tile"=w211) -> ("appended path"=w214:path)  [unwired: 13 in]
            n62 = call "Save module.vi"("Acquisition mode"=FFT_mode."Alazar Spectral", "error in"=w210, "path"=w214, "#A lines"=1250, "#B lines"=1100) -> ("error out"=w209:errorcluster)  [unwired: 6 in]
          }
          frame "Alazar B line" {
            n63 = call "Tile naming.vi"(7:Tile_naming_actions."Increment", "Error In"=w216) -> ("Error Out"=w215:errorcluster)  [unwired: 6 in, 3 out]
            n64 = call "Tile naming.vi"(7:Tile_naming_actions."Export", "Error In"=w215) -> ("Error Out"=w219:errorcluster, "tile"=w220:i32, "slice"=w221:i32)  [unwired: 6 in, 1 out]
            n65 = call "Generate File Name.vi"("slice"=w221, "tile"=w220) -> ("appended path"=w223:path)  [unwired: 13 in]
            n66 = call "Save module.vi"("Acquisition mode"=w218, "error in"=w219, "path"=w223) -> ("error out"=w224:errorcluster)  [unwired: 8 in]
          }
        }
        n67 = call "File log.vi"("action"=T27."Write log", "error in"=w139) -> ("error out"=w138:errorcluster)  [unwired: 9 in]
      }
    }
    n68 = call "Error Message Handler.vi"("Error In"=w114) -> ("Error Out"=w116:errorcluster, "T button?"=w115:bool)  [unwired: 9 in]
    n69 = case shown="True" w115 {
      tunnel: [w122 w128] -> w113
      tunnel: w116 -> [w122 w124]
      frame False {
      }
      frame True {
        n70 = call "Queue Manager.vi"("Queue Name"=QueueNames."Main Saving", "Action"=Queue_Manager_Actions."Flush Queue", "Error In"=w124) -> ("Error Out"=w123:errorcluster)  [unwired: 4 in, 4 out]
        n71 = call "Queue Manager.vi"("Queue Name"=QueueNames."Main Saving", "Action"=Queue_Manager_Actions."Enqueue", "Error In"=w123, "Message Packet Array"=T30[] [{"Message"="Exit", "Parameter"=variant}] ("Message Packet [In]")) -> ("Error Out"=w128:errorcluster)  [unwired: 3 in, 4 out]
      }
    }
  }
  n72 = while {
    shift-right: [w227] -> w16
    shift-left: w2 -> [w236]
    stop <- w237 stop-if-true
    # "Main Scan Processor"
    n73 = call "Queue Manager.vi"("Queue Name"=QueueNames."Main Scan Processor", "timeout in ms (-1)"=-1, "Action"=Queue_Manager_Actions."Dequeue", "Error In"=w236) -> ("Error Out"=w226:errorcluster, "Message Packet [Out]"=w234:T30)  [unwired: 3 in, 3 out]
    n74 = Unbundle(w234) -> ("Message"=w233:string, "Parameter"=w232:variant)
    n75 = case shown="\"Acquire\"" w233 {
      tunnel: w232 -> [_ _ _ _ _ _]
      tunnel: [w238 w240 w246 w248 w265 w272] -> w230
      tunnel: [TRUE _ _ _ _ _] -> w237
      tunnel: w226 -> [w238 w240 w242 w247 w265 w279]
      frame "Exit" {
      }
      frame "Init" {
      }
      frame "Init Hardware" {
        n76 = global write "Main Scan Processor Status.vi" "Busy"(TRUE ("Busy")) -> ()
        n77 = call "Queue Manager.vi"("Queue Name"=QueueNames."Main Scan Processor", "Action"=Queue_Manager_Actions."Enqueue", "Error In"=w242, "Message Packet Array"=T30[] [{"Message"="Init Laser", "Parameter"=variant}, {"Message"="", "Parameter"=variant}, {"Message"="", "Parameter"=variant}, {"Message"="", "Parameter"=variant}, {"Message"="", "Parameter"=variant}, {"Message"="", "Parameter"=variant}, {"Message"="", "Parameter"=variant}]) -> ("Error Out"=w246:errorcluster)  [unwired: 3 in, 4 out]
      }
      frame "Init Laser" {
        n78 = disable-structure shown="Enabled" {
          disable-tunnel: w247 -> [w252 w264]
          disable-tunnel: [w249 w264] -> w248
          frame Disabled {
            n79 = call "Axsun module.vi"("Action"=Axsun_action."Create handle", "error in (no error)"=w252) -> ("error out"=w262:errorcluster)  [unwired: 8 in, 1 out]
            n80 = call "Axsun module.vi"("Action"=Axsun_action."GetControlVersion", "error in (no error)"=w262) -> ("error out"=w261:errorcluster)  [unwired: 8 in, 1 out]
            n81 = call "Axsun module.vi"("Action"=Axsun_action."Start Network Control Interface", "error in (no error)"=w261) -> ("error out"=w260:errorcluster)  [unwired: 8 in, 1 out]
            n82 = call "Axsun module.vi"("Action"=Axsun_action."Get laser handle", "error in (no error)"=w260) -> ("error out"=w259:errorcluster)  [unwired: 8 in, 1 out]
            n83 = call "Axsun module.vi"("Action"=Axsun_action."GetSerialNum", "error in (no error)"=w259) -> ("error out"=w258:errorcluster)  [unwired: 8 in, 1 out]
            n84 = call "Axsun module.vi"("Action"=Axsun_action."GetSystemStatus", "error in (no error)"=w258) -> ("error out"=w250:errorcluster)  [unwired: 8 in, 1 out]
            n85 = call "Axsun module.vi"("Action"=Axsun_action."Laser ON", "error in (no error)"=w250) -> ("error out"=w249:errorcluster)  [unwired: 8 in, 1 out]
          }
          frame Enabled {
          }
        }
      }
      frame "Idle", Default {
        n86 = global write "Main Scan Processor Status.vi" "Busy"(FALSE ("Busy")) -> ()
      }
      frame "Acquire" {
        n87 = call "System Parameters - FGV.vi"("Actions"=FGV_Actions."Get", "Error In"=w279) -> ("Error Out"=w276:errorcluster, "System Parameters [Out]"=w278:T33)  [unwired: 8 in]
        n88 = Unbundle By Name(w278) -> ("Manual Controls.Acquisition mode"=w277:T21)
        n89 = call "File log.vi"("action"=T27."Create file", "error in"=w276) -> ("error out"=w275:errorcluster)  [unwired: 9 in]
        n90 = call "File log.vi"("action"=T27."Write config", "error in"=w275) -> ("error out"=w268:errorcluster)  [unwired: 9 in]
        n91 = call "Save bline to memory1.vi"("action"=Save_Bline_to_Mem_Control."Uninit", "error in"=w268) -> ("error out"=w271:errorcluster)  [unwired: 13 in]
        n92 = call "Save bline to memory2.vi"("action"=Save_Bline_to_Mem_Control."Uninit", "error in"=w271) -> ("error out"=w267:errorcluster)  [unwired: 13 in]
        n93 = case shown="\"Alazar FFT\"" w277 {
          tunnel: [w281 w289 w297 w302 w309 w316] -> w272
          tunnel: w267 -> [w281 w282 w290 w298 w305 w312]
          frame Default {
          }
          frame "Alazar FFT" {
            # "Acquisition mode"
            n94 = global write "Main Scan Processor Status.vi" "Busy"(TRUE ("Busy")) -> ()
            n95 = call "Save bline to memory2.vi"("action"=Save_Bline_to_Mem_Control."PSOCT Spatial buffer Init", "error in"=w282) -> ("error out"=w286:errorcluster)  [unwired: 13 in]
            n96 = call "Save bline to memory1.vi"("action"=Save_Bline_to_Mem_Control."PSOCT Spatial buffer Init", "error in"=w286) -> ("error out"=w284:errorcluster)  [unwired: 13 in]
            n97 = call "Scan Engine.vi"("Message Packet"=T30 {"Message"="Init(Alazar FFT)", "Parameter"=variant}, "Error In"=w284) -> ("Error Out"=w289:errorcluster)  [unwired: 9 in]
          }
          frame "Alazar B line" {
            # "Acquisition mode"
            n98 = global write "Main Scan Processor Status.vi" "Busy"(TRUE ("Busy")) -> ()
            n99 = call "Save bline to memory2.vi"("action"=Save_Bline_to_Mem_Control."PSOCT Spatial buffer Init", "error in"=w290) -> ("error out"=w294:errorcluster)  [unwired: 13 in]
            n100 = call "Save bline to memory1.vi"("action"=Save_Bline_to_Mem_Control."PSOCT Spatial buffer Init", "error in"=w294) -> ("error out"=w293:errorcluster)  [unwired: 13 in]
            n101 = call "Scan Engine.vi"("Message Packet"=T30 {"Message"="Init(Alazar FFT)", "Parameter"=variant}, "Error In"=w293) -> ("Error Out"=w297:errorcluster)  [unwired: 9 in]
          }
          frame "GPU FFT" {
            n102 = call "Save bline to memory2.vi"("action"=Save_Bline_to_Mem_Control."PSOCT Spectral buffer Init", "error in"=w298) -> ("error out"=w303:errorcluster)  [unwired: 13 in]
            n103 = call "Save bline to memory1.vi"("action"=Save_Bline_to_Mem_Control."PSOCT Spectral buffer Init", "error in"=w303) -> ("error out"=w301:errorcluster)  [unwired: 13 in]
            n104 = call "Scan Engine.vi"("Message Packet"=T30 {"Message"="Init(GPU FFT)", "Parameter"=variant}, "Error In"=w301) -> ("Error Out"=w302:errorcluster)  [unwired: 9 in]
          }
          frame "Simulation" {
            n105 = call "Save bline to memory2.vi"("action"=Save_Bline_to_Mem_Control."PSOCT Spectral buffer Init", "error in"=w305) -> ("error out"=w310:errorcluster)  [unwired: 13 in]
            n106 = call "Save bline to memory1.vi"("action"=Save_Bline_to_Mem_Control."PSOCT Spectral buffer Init", "error in"=w310) -> ("error out"=w308:errorcluster)  [unwired: 13 in]
            n107 = call "Scan Engine.vi"("Message Packet"=T30 {"Message"="Init(GPU FFT)", "Parameter"=variant}, "Error In"=w308) -> ("Error Out"=w309:errorcluster)  [unwired: 9 in]
          }
          frame "Alazar Spectral" {
            n108 = call "Save bline to memory2.vi"("action"=Save_Bline_to_Mem_Control."PSOCT Spectral buffer Init", "error in"=w312) -> ("error out"=w317:errorcluster)  [unwired: 13 in]
            n109 = call "Save bline to memory1.vi"("action"=Save_Bline_to_Mem_Control."PSOCT Spectral buffer Init", "error in"=w317) -> ("error out"=w315:errorcluster)  [unwired: 13 in]
            n110 = call "Scan Engine.vi"("Message Packet"=T30 {"Message"="Init(GPU FFT)", "Parameter"=variant}, "Error In"=w315) -> ("Error Out"=w316:errorcluster)  [unwired: 9 in]
          }
        }
      }
    }
    n111 = call "Error Message Handler.vi"("Error In"=w230) -> ("Error Out"=w229:errorcluster, "T button?"=w228:bool)  [unwired: 9 in]
    n112 = case shown="True" w228 {
      tunnel: w229 -> [w319 w321]
      tunnel: [w319 w322] -> w227
      frame False {
      }
      frame True {
        n113 = call "Queue Manager.vi"("Queue Name"=QueueNames."Main Scan Processor", "Action"=Queue_Manager_Actions."Enqueue", "Error In"=w321, "Message Packet Array"=T30[] [{"Message"="Exit", "Parameter"=variant}] ("Message Packet [In]")) -> ("Error Out"=w322:errorcluster)  [unwired: 3 in, 4 out]
      }
    }
  }
  n114 = while "Main Data Processing" {
    shift-right: [w332] -> w9
    shift-left: w2 -> [w336]
    stop <- w328 stop-if-true
    # "Main Processing"
    n115 = call "Queue Manager.vi"("Queue Name"=QueueNames."Main Processing", "Action"=Queue_Manager_Actions."Dequeue", "Error In"=w336) -> ("Error Out"=w327:errorcluster, "Message Packet [Out]"=w330:T30)  [unwired: 4 in, 3 out]
    n116 = Unbundle By Name(w330) -> ("Message"=w325:string, "Parameter"=w326:variant)
    n117 = case shown="\"Process\"" w325 {
      tunnel: [w337 w338 w340 w347 w500 w567] -> w329
      tunnel: [_ TRUE ("Exit") _ _ _ _] -> w328
      tunnel: w327 -> [w337 w338 w340 w345 w498 w565]
      tunnel: w326 -> [_ _ _ _ _ _]
      frame "False", Default {
      }
      frame "Exit" {
      }
      frame "Init" {
      }
      frame "Process" {
        n118 = call "System Parameters - FGV.vi"("Actions"=FGV_Actions."Get", "Error In"=w345) -> ("Error Out"=w344:errorcluster, "System Parameters [Out]"=w341:T33)  [unwired: 8 in]
        n119 = Unbundle By Name(w341) -> ("Manual Controls.Acquisition mode"=w343:T21, "Manual Controls.Save data?"=w342:bool)
        n120 = case shown="\"GPU FFT\"" w343 {
          tunnel: [w348 w355 w384 w413 w442 w471] -> w347
          tunnel: w344 -> [w348 w351 w380 w409 w439 w468]
          tunnel: w342 -> [_ w354 w383 w412 w441 w465]
          frame Default {
          }
          frame "GPU FFT" {
            n121 = call "FGV - Acquisition Status.vi"("Actions"=FGV_Actions."Get", "Error In"=w351) -> ("Error Out"=w350:errorcluster, "mem loc out"=w352:i32)  [unwired: 6 in, 2 out]
            n122 = case shown="2, Default" w352 {
              tunnel: [1 2] -> w349
              frame 2, Default {
              }
              frame 1 {
              }
            }
            n123 = case shown="2" w349 {
              tunnel: [w371 w374 w377] -> w361
              tunnel: w350 -> [w371 w373 w375]
              frame 0, Default {
              }
              frame 1 {
                # "memory block location"
                n124 = call "Save bline to memory1.vi"("action"=Save_Bline_to_Mem_Control."FFT and Save", "error in"=w373) -> ("error out"=w374:errorcluster)  [unwired: 13 in]
              }
              frame 2 {
                # "memory block location"
                n125 = call "Save bline to memory2.vi"("action"=Save_Bline_to_Mem_Control."FFT and Save", "error in"=w375) -> ("error out"=w377:errorcluster)  [unwired: 13 in]
              }
            }
            n126 = case shown="True" w354 {
              tunnel: w361 -> [w364 w366]
              tunnel: [w364 w365] -> w356
              frame False {
                # "do not save"
              }
              frame True {
                # "Save"
                n127 = Build Array(T30 {"Message"="Start", "Parameter"=variant} ("Message Packet Array")) -> (w368:T30[])
                n128 = call "Queue Manager.vi"("Queue Name"=QueueNames."Main Saving", "Action"=Queue_Manager_Actions."Enqueue", "Error In"=w366, "Message Packet Array"=w368) -> ("Error Out"=w365:errorcluster)  [unwired: 3 in, 4 out]
              }
            }
            n129 = Build Array(T30 {"Message"="Update Image", "Parameter"=variant} ("Message Packet Array")) -> (w358:T30[])
            n130 = call "Queue Manager.vi"("Queue Name"=QueueNames."Main Display", "Action"=Queue_Manager_Actions."Enqueue", "Error In"=w356, "Message Packet Array"=w358) -> ("Error Out"=w355:errorcluster)  [unwired: 3 in, 4 out]
          }
          frame "Simulation" {
            n131 = call "FGV - Acquisition Status.vi"("Actions"=FGV_Actions."Get", "Error In"=w380) -> ("Error Out"=w379:errorcluster, "mem loc out"=w381:i32)  [unwired: 6 in, 2 out]
            n132 = case shown="2, Default" w381 {
              tunnel: [1 2] -> w378
              frame 2, Default {
              }
              frame 1 {
              }
            }
            n133 = case shown="1" w378 {
              tunnel: [w400 w403 w406] -> w390
              tunnel: w379 -> [w400 w402 w404]
              frame 0, Default {
              }
              frame 1 {
                # "memory block location"
                n134 = call "Save bline to memory1.vi"("action"=Save_Bline_to_Mem_Control."FFT and Save", "error in"=w402) -> ("error out"=w403:errorcluster)  [unwired: 13 in]
              }
              frame 2 {
                # "memory block location"
                n135 = call "Save bline to memory2.vi"("action"=Save_Bline_to_Mem_Control."FFT and Save", "error in"=w404) -> ("error out"=w406:errorcluster)  [unwired: 13 in]
              }
            }
            n136 = case shown="True" w383 {
              tunnel: w390 -> [w393 w395]
              tunnel: [w393 w394] -> w385
              frame False {
                # "do not save"
              }
              frame True {
                # "Save"
                n137 = Build Array(T30 {"Message"="Start", "Parameter"=variant} ("Message Packet Array")) -> (w397:T30[])
                n138 = call "Queue Manager.vi"("Queue Name"=QueueNames."Main Saving", "Action"=Queue_Manager_Actions."Enqueue", "Error In"=w395, "Message Packet Array"=w397) -> ("Error Out"=w394:errorcluster)  [unwired: 3 in, 4 out]
              }
            }
            n139 = Build Array(T30 {"Message"="Update Image", "Parameter"=variant} ("Message Packet Array")) -> (w387:T30[])
            n140 = call "Queue Manager.vi"("Queue Name"=QueueNames."Main Display", "Action"=Queue_Manager_Actions."Enqueue", "Error In"=w385, "Message Packet Array"=w387) -> ("Error Out"=w384:errorcluster)  [unwired: 3 in, 4 out]
          }
          frame "Alazar Spectral" {
            n141 = call "FGV - Acquisition Status.vi"("Actions"=FGV_Actions."Get", "Error In"=w409) -> ("Error Out"=w408:errorcluster, "mem loc out"=w410:i32)  [unwired: 6 in, 2 out]
            n142 = case shown="1" w410 {
              tunnel: [1 2] -> w407
              frame 2, Default {
              }
              frame 1 {
              }
            }
            n143 = case shown="1" w407 {
              tunnel: [w429 w432 w435] -> w419
              tunnel: w408 -> [w429 w431 w433]
              frame 0, Default {
              }
              frame 1 {
                # "memory block location"
                n144 = call "Save bline to memory1.vi"("action"=Save_Bline_to_Mem_Control."Alazar Spectral Save", "error in"=w431) -> ("error out"=w432:errorcluster)  [unwired: 13 in]
              }
              frame 2 {
                # "memory block location"
                n145 = call "Save bline to memory2.vi"("action"=Save_Bline_to_Mem_Control."Alazar Spectral Save", "error in"=w433) -> ("error out"=w435:errorcluster)  [unwired: 13 in]
              }
            }
            n146 = case shown="True" w412 {
              tunnel: w419 -> [w422 w424]
              tunnel: [w422 w423] -> w414
              frame False {
                # "do not save"
              }
              frame True {
                # "Save"
                n147 = Build Array(T30 {"Message"="Start", "Parameter"=variant} ("Message Packet Array")) -> (w426:T30[])
                n148 = call "Queue Manager.vi"("Queue Name"=QueueNames."Main Saving", "Action"=Queue_Manager_Actions."Enqueue", "Error In"=w424, "Message Packet Array"=w426) -> ("Error Out"=w423:errorcluster)  [unwired: 3 in, 4 out]
              }
            }
            n149 = Build Array(T30 {"Message"="Update Image", "Parameter"=variant} ("Message Packet Array")) -> (w416:T30[])
            n150 = call "Queue Manager.vi"("Queue Name"=QueueNames."Main Display", "Action"=Queue_Manager_Actions."Enqueue", "Error In"=w414, "Message Packet Array"=w416) -> ("Error Out"=w413:errorcluster)  [unwired: 3 in, 4 out]
          }
          frame "Alazar FFT" {
            n151 = call "FGV - Acquisition Status.vi"("Actions"=FGV_Actions."Get", "Error In"=w439) -> ("Error Out"=w438:errorcluster, "mem loc out"=w437:i32)  [unwired: 6 in, 2 out]
            n152 = case shown="1" w437 {
              tunnel: [1 2] -> w436
              frame 2, Default {
              }
              frame 1 {
              }
            }
            n153 = case shown="1" w436 {
              tunnel: [w458 w461 w464] -> w448
              tunnel: w438 -> [w458 w460 w463]
              frame 0, Default {
              }
              frame 1 {
                # "memory block location"
                n154 = call "Save bline to memory1.vi"("action"=Save_Bline_to_Mem_Control."Save(PSOCT)", "error in"=w460) -> ("error out"=w461:errorcluster)  [unwired: 13 in]
              }
              frame 2 {
                # "memory block location"
                n155 = call "Save bline to memory2.vi"("action"=Save_Bline_to_Mem_Control."Save(PSOCT)", "error in"=w463) -> ("error out"=w464:errorcluster)  [unwired: 13 in]
              }
            }
            n156 = case shown="True" w441 {
              tunnel: w448 -> [w451 w453]
              tunnel: [w451 w452] -> w443
              frame False {
                # "do not save"
              }
              frame True {
                # "Save"
                n157 = Build Array(T30 {"Message"="Start", "Parameter"=variant} ("Message Packet Array")) -> (w455:T30[])
                n158 = call "Queue Manager.vi"("Queue Name"=QueueNames."Main Saving", "Action"=Queue_Manager_Actions."Enqueue", "Error In"=w453, "Message Packet Array"=w455) -> ("Error Out"=w452:errorcluster)  [unwired: 3 in, 4 out]
              }
            }
            n159 = Build Array(T30 {"Message"="Update Image", "Parameter"=variant} ("Message Packet Array")) -> (w445:T30[])
            n160 = call "Queue Manager.vi"("Queue Name"=QueueNames."Main Display", "Action"=Queue_Manager_Actions."Enqueue", "Error In"=w443, "Message Packet Array"=w445) -> ("Error Out"=w442:errorcluster)  [unwired: 3 in, 4 out]
          }
          frame "Alazar B line" {
            n161 = call "FGV - Acquisition Status.vi"("Actions"=FGV_Actions."Get", "Error In"=w468) -> ("Error Out"=w467:errorcluster, "mem loc out"=w469:i32)  [unwired: 6 in, 2 out]
            n162 = case shown="2, Default" w469 {
              tunnel: [1 2] -> w466
              frame 2, Default {
              }
              frame 1 {
              }
            }
            n163 = case shown="1" w466 {
              tunnel: [w487 w490 w493] -> w477
              tunnel: w467 -> [w487 w489 w492]
              frame 0, Default {
              }
              frame 1 {
                # "memory block location"
                n164 = call "Save bline to memory1.vi"("action"=Save_Bline_to_Mem_Control."Save(PSOCT)", "error in"=w489) -> ("error out"=w490:errorcluster)  [unwired: 13 in]
              }
              frame 2 {
                # "memory block location"
                n165 = call "Save bline to memory2.vi"("action"=Save_Bline_to_Mem_Control."Save(PSOCT)", "error in"=w492) -> ("error out"=w493:errorcluster)  [unwired: 13 in]
              }
            }
            n166 = case shown="True" w465 {
              tunnel: w477 -> [w480 w482]
              tunnel: [w480 w481] -> w472
              frame False {
                # "do not save"
              }
              frame True {
                # "Save"
                n167 = Build Array(T30 {"Message"="Start", "Parameter"=variant} ("Message Packet Array")) -> (w484:T30[])
                n168 = call "Queue Manager.vi"("Queue Name"=QueueNames."Main Saving", "Action"=Queue_Manager_Actions."Enqueue", "Error In"=w482, "Message Packet Array"=w484) -> ("Error Out"=w481:errorcluster)  [unwired: 3 in, 4 out]
              }
            }
            n169 = Build Array(T30 {"Message"="Update Image", "Parameter"=variant} ("Message Packet Array")) -> (w474:T30[])
            n170 = call "Queue Manager.vi"("Queue Name"=QueueNames."Main Display", "Action"=Queue_Manager_Actions."Enqueue", "Error In"=w472, "Message Packet Array"=w474) -> ("Error Out"=w471:errorcluster)  [unwired: 3 in, 4 out]
          }
        }
      }
      frame "Skip" {
        n171 = call "System Parameters - FGV.vi"("Actions"=FGV_Actions."Get", "Error In"=w498) -> ("Error Out"=w497:errorcluster, "System Parameters [Out]"=w494:T33)  [unwired: 8 in]
        n172 = Unbundle By Name(w494) -> ("Manual Controls.Acquisition mode"=w496:T21, "Manual Controls.Save data?"=w495:bool)
        n173 = case shown="\"Simulation\"" w496 {
          tunnel: [w501 w502 w513 w523 w533 w543 w553] -> w500
          tunnel: w497 -> [w501 w503 w512 w522 w532 w542 w552]
          tunnel: w495 -> [_ w504 w514 w524 w534 w544 w554]
          frame Default {
          }
          frame "GPU FFT" {
            n174 = case shown="True" w504 {
              tunnel: w503 -> [w505 w507]
              tunnel: [w505 w506] -> w502
              frame False {
                # "do not save"
              }
              frame True {
                # "Save"
                n175 = Build Array(T30 {"Message"="Start", "Parameter"=variant} ("Message Packet Array")) -> (w509:T30[])
                n176 = call "Queue Manager.vi"("Queue Name"=QueueNames."Main Saving", "Action"=Queue_Manager_Actions."Enqueue", "Error In"=w507, "Message Packet Array"=w509) -> ("Error Out"=w506:errorcluster)  [unwired: 3 in, 4 out]
              }
            }
          }
          frame "Save all" {
            n177 = case shown="True" w514 {
              tunnel: w512 -> [w515 w517]
              tunnel: [w515 w516] -> w513
              frame False {
                # "do not save"
              }
              frame True {
                # "Save"
                n178 = Build Array(T30 {"Message"="Start", "Parameter"=variant} ("Message Packet Array")) -> (w519:T30[])
                n179 = call "Queue Manager.vi"("Queue Name"=QueueNames."Main Saving", "Action"=Queue_Manager_Actions."Enqueue", "Error In"=w517, "Message Packet Array"=w519) -> ("Error Out"=w516:errorcluster)  [unwired: 3 in, 4 out]
              }
            }
          }
          frame "Simulation" {
            n180 = case shown="True" w524 {
              tunnel: w522 -> [w525 w527]
              tunnel: [w525 w526] -> w523
              frame False {
                # "do not save"
              }
              frame True {
                # "Save"
                n181 = Build Array(T30 {"Message"="Start", "Parameter"=variant} ("Message Packet Array")) -> (w529:T30[])
                n182 = call "Queue Manager.vi"("Queue Name"=QueueNames."Main Saving", "Action"=Queue_Manager_Actions."Enqueue", "Error In"=w527, "Message Packet Array"=w529) -> ("Error Out"=w526:errorcluster)  [unwired: 3 in, 4 out]
              }
            }
          }
          frame "Alazar Spectral" {
            n183 = case shown="True" w534 {
              tunnel: w532 -> [w535 w537]
              tunnel: [w535 w536] -> w533
              frame False {
                # "do not save"
              }
              frame True {
                # "Save"
                n184 = Build Array(T30 {"Message"="Start", "Parameter"=variant} ("Message Packet Array")) -> (w539:T30[])
                n185 = call "Queue Manager.vi"("Queue Name"=QueueNames."Main Saving", "Action"=Queue_Manager_Actions."Enqueue", "Error In"=w537, "Message Packet Array"=w539) -> ("Error Out"=w536:errorcluster)  [unwired: 3 in, 4 out]
              }
            }
          }
          frame "Alazar FFT" {
            n186 = case shown="False" w544 {
              tunnel: w542 -> [w545 w547]
              tunnel: [w545 w546] -> w543
              frame False {
                # "do not save"
              }
              frame True {
                # "Save"
                n187 = Build Array(T30 {"Message"="Start", "Parameter"=variant} ("Message Packet Array")) -> (w549:T30[])
                n188 = call "Queue Manager.vi"("Queue Name"=QueueNames."Main Saving", "Action"=Queue_Manager_Actions."Enqueue", "Error In"=w547, "Message Packet Array"=w549) -> ("Error Out"=w546:errorcluster)  [unwired: 3 in, 4 out]
              }
            }
          }
          frame "Alazar B line" {
            n189 = case shown="True" w554 {
              tunnel: w552 -> [w555 w557]
              tunnel: [w555 w556] -> w553
              frame False {
                # "do not save"
              }
              frame True {
                # "Save"
                n190 = Build Array(T30 {"Message"="Start", "Parameter"=variant} ("Message Packet Array")) -> (w559:T30[])
                n191 = call "Queue Manager.vi"("Queue Name"=QueueNames."Main Saving", "Action"=Queue_Manager_Actions."Enqueue", "Error In"=w557, "Message Packet Array"=w559) -> ("Error Out"=w556:errorcluster)  [unwired: 3 in, 4 out]
              }
            }
          }
        }
      }
      frame "Average" {
        n192 = call "System Parameters - FGV.vi"("Actions"=FGV_Actions."Get", "Error In"=w565) -> ("Error Out"=w564:errorcluster, "System Parameters [Out]"=w562:T33)  [unwired: 8 in]
        n193 = Unbundle By Name(w562) -> ("Manual Controls.Acquisition mode"=w563:T21)
        n194 = case shown="\"Alazar FFT\", Default" w563 {
          tunnel: [w568] -> w567
          tunnel: w564 -> [w572]
          frame "Alazar FFT", Default {
            n195 = call "FGV - Acquisition Status.vi"("Actions"=FGV_Actions."Get", "Error In"=w572) -> ("Error Out"=w571:errorcluster, "mem loc out"=w570:i32)  [unwired: 6 in, 2 out]
            n196 = case shown="1" w570 {
              tunnel: [1 2] -> w569
              frame 2, Default {
              }
              frame 1 {
              }
            }
            n197 = case shown="1" w569 {
              tunnel: [w576 w579 w582] -> w568
              tunnel: w571 -> [w576 w578 w581]
              frame 0, Default {
              }
              frame 1 {
                # "memory block location"
                n198 = call "Save bline to memory1.vi"("action"=Save_Bline_to_Mem_Control."Average", "error in"=w578) -> ("error out"=w579:errorcluster)  [unwired: 13 in]
              }
              frame 2 {
                # "memory block location"
                n199 = call "Save bline to memory2.vi"("action"=Save_Bline_to_Mem_Control."Average", "error in"=w581) -> ("error out"=w582:errorcluster)  [unwired: 13 in]
              }
            }
          }
        }
      }
    }
    n200 = call "Error Message Handler.vi"("Error In"=w329) -> ("Error Out"=w333:errorcluster, "T button?"=w331:bool)  [unwired: 9 in]
    n201 = case shown="False" w331 {
      tunnel: w333 -> [w583 w585]
      tunnel: [w583 w586] -> w332
      frame False {
      }
      frame True {
        n202 = call "Queue Manager.vi"("Queue Name"=QueueNames."Main Processing", "Action"=Queue_Manager_Actions."Enqueue", "Error In"=w585, "Message Packet Array"=T30[] [{"Message"="Exit", "Parameter"=variant}] ("Message Packet [In]")) -> ("Error Out"=w586:errorcluster)  [unwired: 3 in, 4 out]
      }
    }
  }
  n203 = while {
    shift-right: [w590] -> w21
    shift-left: w2 -> [w599]
    stop <- w600 stop-if-true
    # "Main GUI"
    n204 = call "Queue Manager.vi"("Queue Name"=QueueNames."Main GUI", "Action"=Queue_Manager_Actions."Dequeue", "Error In"=w599) -> ("Error Out"=w597:errorcluster, "Message Packet [Out]"=w596:T30)  [unwired: 4 in, 3 out]
    n205 = Unbundle(w596) -> ("Message"=w593:string, "Parameter"=w595:variant)
    n206 = case shown="\"Wait for User Input\"" w593 {
      tunnel: w597 -> [w615 w667 w673 w699 w719 w736 w749 w1064 w1085]
      tunnel: w595 -> [_ _ _ _ _ _ _ _ _]
      tunnel: [w614 w663 w669 w691 w715 w734 w750 w1057 w1085] -> w589
      tunnel: [_ _ _ _ _ _ _ TRUE _] -> w600
      frame "Init" {
        n207 = call "Queue Manager.vi"("Queue Name"=QueueNames."Main GUI", "Action"=Queue_Manager_Actions."Enqueue", "Error In"=w615, "Message Packet Array"=T30[] [{"Message"="Init Variables", "Parameter"=variant}, {"Message"="Set Front Panel", "Parameter"=variant}, {"Message"="Update User Settings", "Parameter"=variant}, {"Message"="Configure Hardware", "Parameter"=variant}, {"Message"="Wait for Complete", "Parameter"=variant}, {"Message"="Wait for User Input", "Parameter"=variant}]) -> ("Error Out"=w614:errorcluster)  [unwired: 3 in, 4 out]
      }
      frame "Init Variables" {
        n208 = call "Status Queue.vi"("Action"=Queue_Manager_Actions."Enqueue", "Error In"=w667, "Status Message [In]"="Initializing Variables...") -> ("Error Out"=w662:errorcluster)  [unwired: 7 in, 1 out]
        n209 = call "Alazar_simulate.vi"("Enum"=enum16{"init", "output"}."init") -> ()  [unwired: 10 in, 1 out]
        n210 = control-ref of="This VI"() -> (w665:refnum<vi>)
        n211 = call "Defer Panel Updates.vi"("Action"=enum16{"Init", "Freeze", "Unfreeze"}."Init", "Error In"=w662, "reference"=w665) -> ("Error Out"=w652:errorcluster)  [unwired: 8 in]
        n212 = call "Image Queue.vi"("Action"=Queue_Manager_Actions."Init", "Error In"=w652) -> ("Error Out"=w618:errorcluster)  [unwired: 8 in, 1 out]
        n213 = call "2P power status.vi"("Actions"=FGV_Actions."Init", "Error In"=w618) -> ("Error Out"=w619:errorcluster)  [unwired: 7 in, 2 out]
        n214 = call "System Parameters - FGV.vi"("Actions"=FGV_Actions."Init", "Error In"=w619) -> ("Error Out"=w632:errorcluster)  [unwired: 8 in, 1 out]
        n215 = call "Display Data Queue 32bit.vi"("max queue size (-1, unlimited)"=5, "Action"=Queue_Manager_Actions."Init", "error in (no error)"=w632) -> ("error out"=w631:errorcluster)  [unwired: 5 in, 3 out]
        n216 = call "Spatial Data Queue 32bit.vi"("max queue size (-1, unlimited)"=5, "Action"=Queue_Manager_Actions."Init", "error in (no error)"=w631) -> ("error out"=w630:errorcluster)  [unwired: 5 in, 3 out]
        n217 = call "Tile naming.vi"(7:Tile_naming_actions."Init", "Error In"=w630) -> ("Error Out"=w621:errorcluster)  [unwired: 6 in, 3 out]
        n218 = call "User Input block.vi"("action"=Pause_action."Init", "error in"=w621, "Pause!"=FALSE) -> ("error out"=w625:errorcluster)  [unwired: 7 in, 1 out]
        n219 = call "Display Data Queue 16bit.vi"("max queue size (-1, unlimited)"=5, "Action"=Queue_Manager_Actions."Init", "error in (no error)"=w625) -> ("error out"=w646:errorcluster)  [unwired: 5 in, 3 out]
        n220 = call "refnum variable.vi"("action"=refnum_control."Init", "error in (no error)"=w621, "reference in"="Attenuator") -> ()  [unwired: 7 in, 2 out]
        n221 = call "Spectral Save Queue.vi"("max queue size (-1, unlimited)"=5, "Action"=Queue_Manager_Actions."Init", "error in (no error)"=w646) -> ("error out"=w645:errorcluster)  [unwired: 5 in, 3 out]
        n222 = call "Save Data Queue.vi"("max queue size (-1, unlimited)"=5, "Action"=Queue_Manager_Actions."Init", "error in (no error)"=w645) -> ("error out"=w638:errorcluster)  [unwired: 5 in, 3 out]
        n223 = call "retardance queue.vi"("max queue size (-1, unlimited)"=5, "Action"=Queue_Manager_Actions."Init", "error in (no error)"=w638) -> ("error out"=w634:errorcluster)  [unwired: 5 in, 3 out]
        n224 = call "Pause.vi"("action"=Pause_action."Init", "error in"=w634) -> ("error out"=w635:errorcluster)  [unwired: 8 in, 1 out]
        n225 = call "Read Config from File.vi"("error in (no error)"=w635) -> ("error out"=w642:errorcluster, "System Parameters"=w617:T33)  [unwired: 9 in]
        n226 = call "System Parameters - FGV.vi"("Actions"=FGV_Actions."Set", "Error In"=w642, "System Parameters [In]"=w617) -> ("Error Out"=w647:errorcluster)  [unwired: 7 in, 1 out]
        n227 = control-ref of="Imaging Parameter"() -> (w655:refnum<vi>)
        n228 = call "Set Front Panel Custom Image Size Cluster Control.vi"("error in (no error)"=w647, "Enable/Disable"=FALSE, "Init"=TRUE, "Cluster Ref In"=w655) -> ("error IO"=w657:errorcluster)  [unwired: 7 in]
        n229 = call "FGV - Acquisition Status.vi"("Actions"=FGV_Actions."Init", "Error In"=w657) -> ("Error Out"=w663:errorcluster, "Scan Type [Out]"=w658:T6)  [unwired: 6 in, 2 out]
        n230 = local write "Scan Type"(w658) -> ()
      }
      frame "Set Front Panel" {
        n231 = call "Status Queue.vi"("Action"=Queue_Manager_Actions."Enqueue", "Error In"=w673, "Status Message [In]"="Setting Front Panel Controls...") -> ("Error Out"=w674:errorcluster)  [unwired: 7 in, 1 out]
        n232 = call "Defer Panel Updates.vi"("Action"=enum16{"Init", "Freeze", "Unfreeze"}."Freeze", "Error In"=w674) -> ("Error Out"=w681:errorcluster)  [unwired: 9 in]
        n233 = call "FGV - Acquisition Status.vi"("Actions"=FGV_Actions."Get", "Error In"=w681) -> ("Error Out"=w678:errorcluster, "Scan Type [Out]"=w677:T6)  [unwired: 6 in, 2 out]
        n234 = case "Acquiring?" shown="False" FALSE {
          tunnel: [w685 w690] -> w679
          tunnel: w678 -> [w686 w690]
          tunnel: w677 -> [w684 _]
          frame False {
            # "Non-Acquiring FP States"
            n235 = disable-structure shown="Enabled" {
              disable-tunnel: w686 -> [w689 _]
              disable-tunnel: [w688 _] -> w685
              disable-tunnel: w684 -> [w687 _]
              frame Disabled {
                n236 = call "Set Main GUI for Different Acquire States.vi"("Error In"=w689, "Scan Type [Out]"=w687) -> ("Error Out"=w688:errorcluster)  [unwired: 9 in]
              }
              frame Enabled {
              }
            }
          }
          frame True {
            # "Acquiring FP States"
          }
        }
        n237 = call "Defer Panel Updates.vi"("Action"=enum16{"Init", "Freeze", "Unfreeze"}."Unfreeze", "Error In"=w679) -> ("Error Out"=w670:errorcluster)  [unwired: 9 in]
        n238 = call "Status Queue.vi"("Action"=Queue_Manager_Actions."Enqueue", "Error In"=w670, "Status Message [In]"="Finished Setting Front Panel.") -> ("Error Out"=w669:errorcluster)  [unwired: 7 in, 1 out]
      }
      frame "Update User Settings" {
        n239 = disable-structure shown="Enabled" {
          disable-tunnel: [Queue_Manager_Actions."Enqueue" ("Action") Queue_Manager_Actions."Enqueue" ("Action")] -> w693
          frame Enabled {
            n240 = call "System Parameters - FGV.vi"("Actions"=FGV_Actions."Get") -> ("System Parameters [Out]"=w712:T33)  [unwired: 9 in, 1 out]
            n241 = Unbundle By Name(w712) -> ("Optical Parameters"=w710:T2, "Vibratome"=w709:T15, "Table Stages"=w708:T23, "Imaging Parameter"=w707:T4, "Galvo HW Parameters"=w706:T42, "Alazar parameters"=w705:T7, "Mosaic Paramter"=w704:T43, "Z stage setting"=w703:T14, "Manual Controls"=w702:T19, "Attenuator"=w701:T18)
            n242 = local write "Galvo HW Parameters"(w706) -> ()
            n243 = local write "Vibratome"(w709) -> ()
            n244 = local write "Alazar parameters"(w705) -> ()
            n245 = local write "Imaging Parameter"(w707) -> ()
            n246 = local write "Optical Parameters"(w710) -> ()
            n247 = local write "Table Stages"(w708) -> ()
            n248 = local write "Manual Controls"(w702) -> ()
            n249 = local write "Mosaic Paramter"(w704) -> ()
            n250 = local write "Attenuator"(w701) -> ()
            n251 = local write "Z stage settings"(w703) -> ()
          }
          frame Disabled {
          }
        }
        n252 = call "Status Queue.vi"("Action"=w693, "Error In"=w699, "Status Message [In]"="Loading User Settings...") -> ("Error Out"=w697:errorcluster)  [unwired: 7 in, 1 out]
        n253 = call "Defer Panel Updates.vi"("Action"=enum16{"Init", "Freeze", "Unfreeze"}."Freeze", "Error In"=w697) -> ("Error Out"=w692:errorcluster)  [unwired: 9 in]
        n254 = call "Set Front Panel Custom Image Size Cluster Control.vi"("error in (no error)"=w692, "Enable/Disable"=TRUE) -> ("error IO"=w695:errorcluster)  [unwired: 9 in]
        n255 = call "Defer Panel Updates.vi"("Action"=enum16{"Init", "Freeze", "Unfreeze"}."Unfreeze", "Error In"=w695) -> ("Error Out"=w691:errorcluster)  [unwired: 9 in]
      }
      frame "Configure Hardware" {
        n256 = call "Status Queue.vi"("Action"=Queue_Manager_Actions."Enqueue", "Error In"=w719, "Status Message [In]"="Initializing Hardware...") -> ("Error Out"=w718:errorcluster)  [unwired: 7 in, 1 out]
        n257 = Build Array(T30 {"Message"="Init Hardware", "Parameter"=variant} ("Message Packet [In]")) -> (w716:T30[])
        n258 = call "Queue Manager.vi"("Queue Name"=QueueNames."Main Scan Processor", "Action"=Queue_Manager_Actions."Enqueue", "Error In"=w718, "Message Packet Array"=w716) -> ("Error Out"=w715:errorcluster)  [unwired: 3 in, 4 out]
      }
      frame "Wait for Complete" {
        n259 = call "TickTock.vi"("Error In"=w736) -> ("Error Out"=w732:errorcluster, "Current Time (Out)"=w731:timestamp)  [unwired: 8 in, 1 out]
        n260 = while {
          shift-right: [w739] -> w733
          shift-left: w732 -> [w747]
          tunnel: w731 -> [w746]
          tunnel: [w737] -> w730
          stop <- w738 stop-if-true
          n261 = call "Inline Wait.vi"("Error In"=w747, "milliseconds to wait"=u32 100) -> ("Error Out"=w743:errorcluster)  [unwired: 9 in]
          n262 = call "TickTock.vi"("Error In"=w743, "Current Time (In)"=w746) -> ("Error Out"=w739:errorcluster, "dt"=w745:dbl)  [unwired: 7 in, 1 out]
          n263 = Greater?(x=60000.0, y=w745) -> (0:w737:bool)
          n264 = global read "Main Scan Processor Status.vi" "Busy"() -> (w741:bool)
          n265 = Not(x=w741) -> (.not. x?=w740:bool)
          n266 = Or(x=w737, y=w740) -> (x .or. y?=w738:bool)
        }
        n267 = Concatenate Strings("Completed." ("Status Message [In]"), "\r\n", " Stephan? What are you doing Stephan?" ("Status Message [In]")) -> (w724:string)
        n268 = Select(t=w724, s=w730, f="Operation timed out." ("Status Message [In]")) -> (s? t:f=w728:string)
        n269 = call "Status Queue.vi"("Action"=Queue_Manager_Actions."Enqueue", "Error In"=w733, "Status Message [In]"=w728) -> ("Error Out"=w734:errorcluster)  [unwired: 7 in, 1 out]
      }
      frame "Wait for User Input" {
        n270 = event shown="[0] Timeout" {
          selector: _ -> [_ _ _ _ _ _ _ _ _ _ _]
          dyn-events: _ -> [_ _ _ _ _ _ _ _ _ _ _]
          timeout: 100 -> [_ _ _ _ _ _ _ _ _ _ _]
          tunnel: [w769 w818 w863 w894 w930 w982 w988 w1000 w1016 w1029 w1045] -> w750
          tunnel: w749 -> [w775 w819 w870 w895 w931 w971 w993 w1002 w1013 w1033 w1046]
          event Timeout {
            n271 = event-data() -> ()  [unwired: 1 in, 3 out]
            n272 = Unbundle By Name("Imaging Parameter") -> ("Pixel Dwell Time [Clock Cycles]"=w758:u16, "Custom Size.X"=w755:u16, "Custom Size.Y"=w756:u16, "Line Averages"=w757:u16)
            n273 = disable-structure shown="Enabled" {
              disable-tunnel: w775 -> [w811 w817]
              disable-tunnel: [w810 w817] -> w767
              frame Disabled {
                n274 = while {
                  tunnel: w811 -> [w812]
                  tunnel: [w815] -> w810
                  stop <- w814 stop-if-true
                  n275 = call "User Input block.vi"("action"=Pause_action."get", "error in"=w812) -> ("error out"=w815:errorcluster, "Pause?"=w813:bool)  [unwired: 8 in]
                  n276 = Not(x=w813) -> (.not. x?=w814:bool)
                }
              }
              frame Enabled {
              }
            }
            n277 = To Unsigned Quad Integer(1:w755) -> (0:w753:u64)
            n278 = To Unsigned Quad Integer(1:w758) -> (0:w754:u64)
            n279 = To Unsigned Quad Integer(1:w756) -> (0:w752:u64)
            n280 = To Unsigned Quad Integer(1:w757) -> (0:w751:u64)
            n281 = Compound Arithmetic op=MULTIPLY(w754, w753, w752, w751) -> (w761:u64)
            n282 = Compound Arithmetic op=MULTIPLY(w754, w753) -> (w759:u64)
            n283 = Bundle By Name(cluster="Alazar parameters", "Acq Settings.Records Per Buffer"=w759, "Acq Settings.Records Count (Records/Acq)"=w761) -> (w760:T7)
            n284 = call "2P power2angle convertor.vi"("Error In"=w767, "power(mW)"="attenuator power(mW)") -> ("Error Out"=w766:errorcluster, "angle"=→"attenuator angle":dbl)  [unwired: 8 in]
            n285 = call "System Parameters - FGV.vi"("Actions"=FGV_Actions."Get", "Error In"=w766) -> ("Error Out"=w783:errorcluster, "System Parameters [Out]"=w804:T33)  [unwired: 8 in]
            n286 = Bundle By Name(cluster=w804, "Vibratome"="Vibratome", "Optical Parameters"="Optical Parameters", "Imaging Parameter"="Imaging Parameter", "Galvo HW Parameters"="Galvo HW Parameters", "Alazar parameters"=w760, "Table Stages"="Table Stages", "Mosaic Paramter"="Mosaic Paramter", "Z stage setting"="Z stage settings", "Manual Controls"="Manual Controls", "Attenuator"="Attenuator") -> (w805:T33)
            n287 = call "System Parameters - FGV.vi"("Actions"=FGV_Actions."Set", "Error In"=w783, "System Parameters [In]"=w805) -> ("Error Out"=w799:errorcluster)  [unwired: 7 in, 1 out]
            n288 = call "XYZ Table Stage Module.vi"("Set/Get"=Set_Get_Controls."Get", "Action"=Motion_Translation_Module_Control2."Position", "Error In"=w783, "Axis"=enum16{"X Axis", "Y Axis", "Z Axis"}."X Axis", "Table Stages"="Table Stages") -> ("Error Out"=w785:errorcluster, "Table Stages [out]"=w787:T23)  [unwired: 5 in]
            n289 = call "XYZ Table Stage Module.vi"("Set/Get"=Set_Get_Controls."Get", "Action"=Motion_Translation_Module_Control2."Position", "Error In"=w785, "Axis"=enum16{"X Axis", "Y Axis", "Z Axis"}."Y Axis", "Table Stages"=w787) -> ("Error Out"=w784:errorcluster, "Table Stages [out]"=w786:T23)  [unwired: 5 in]
            n290 = call "Queue Manager.vi"("Queue Name"=QueueNames."Main GUI", "Action"=Queue_Manager_Actions."Enqueue", "Error In"=w799, "Message Packet Array"=T30[] [{"Message"="Wait for User Input", "Parameter"=variant}]) -> ("Error Out"=w770:errorcluster)  [unwired: 3 in, 4 out]
            n291 = call "XYZ Table Stage Module.vi"("Set/Get"=Set_Get_Controls."Get", "Action"=Motion_Translation_Module_Control2."Position", "Error In"=w784, "Axis"=enum16{"X Axis", "Y Axis", "Z Axis"}."Z Axis", "Table Stages"=w786) -> ("Table Stages [out]"=w782:T23)  [unwired: 5 in, 1 out]
            n292 = Unbundle By Name(w782) -> ("X Stage.Position"=w780:dbl, "Y Stage.Position"=w779:dbl, "Z Stage.Position"=w778:dbl)
            n293 = call "Queue Manager.vi"("Queue Name"=QueueNames."Main Display", "Action"=Queue_Manager_Actions."Enqueue", "Error In"=w770, "Message Packet Array"=T30[] [{"Message"="Update Status", "Parameter"=variant}]) -> ("Error Out"=w769:errorcluster)  [unwired: 3 in, 4 out]
            n294 = Bundle By Name(cluster=cluster{"X":dbl, "Y":dbl, "Z":dbl} {"X"=0.0, "Y"=0.0, "Z"=0.0} ("Current Position out 2"), "X"=w780, "Y"=w779, "Z"=w778) -> (→"Current Position out":cluster{"X":dbl, "Y":dbl, "Z":dbl})
          }
          event Value Change {
            n295 = event-data() -> ("NewVal"=w820:bool)  [unwired: 1 in, 5 out]
            n296 = case shown="True" w820 {
              tunnel: w819 -> [w822 w833]
              tunnel: [w821 w831] -> w818
              frame False {
                n297 = call "Queue Manager.vi"("Queue Name"=QueueNames."Main GUI", "Action"=Queue_Manager_Actions."Enqueue", "Error In"=w822, "Message Packet Array"=T30[] [{"Message"="Wait for User Input", "Parameter"=variant}]) -> ("Error Out"=w821:errorcluster)  [unwired: 3 in, 4 out]
              }
              frame True {
                n298 = call "System Parameters - FGV.vi"("Actions"=FGV_Actions."Get", "Error In"=w833) -> ("Error Out"=w834:errorcluster, "System Parameters [Out]"=w832:T33)  [unwired: 8 in]
                n299 = Unbundle By Name(w832) -> ("Table Stages.X Stage.Position"=w827:dbl, "Table Stages"=w828:T23)
                n300 = call "Queue Manager.vi"("Queue Name"=QueueNames."Main GUI", "Action"=Queue_Manager_Actions."Enqueue", "Error In"=w834, "Message Packet Array"=T30[] [{"Message"="Wait for User Input", "Parameter"=variant}]) -> ("Error Out"=w830:errorcluster)  [unwired: 3 in, 4 out]
                n301 = call "X stage safety.vi"("new position"=w827, "Error In"=w830, "Table Stages"=w828) -> ("Error Out"=w829:errorcluster, "crash?"=w826:bool)  [unwired: 7 in]
                n302 = case shown="True" w826 {
                  tunnel: w829 -> [w839 w845]
                  tunnel: [w839 w844] -> w831
                  tunnel: w828 -> [_ w843]
                  frame True {
                    n303 = Two Button Dialog(message="Warning: about to crash!!! Movement invalid" ("T button name (\"OK\")"), 1:"Abort" ("F button name (\"Cancel\")"), 2:"Abort" ("T button name (\"OK\")")) -> ()  [unwired: 1 out]
                  }
                  frame False {
                    n304 = call "XYZ Table Stage Module.vi"("Set/Get"=Set_Get_Controls."Set", "Action"=Motion_Translation_Module_Control2."Velocity/Accel", "Error In"=w845, "Axis"=enum16{"X Axis", "Y Axis", "Z Axis"}."X Axis", "Table Stages"=w843) -> ("Error Out"=w848:errorcluster, "Table Stages [out]"=w849:T23)  [unwired: 5 in]
                    n305 = call "XYZ Table Stage Module.vi"("Set/Get"=Set_Get_Controls."Set", "Action"=Motion_Translation_Module_Control2."Position", "Error In"=w848, "Axis"=enum16{"X Axis", "Y Axis", "Z Axis"}."X Axis", "Table Stages"=w849) -> ("Error Out"=w844:errorcluster)  [unwired: 5 in, 1 out]
                  }
                }
              }
            }
          }
          event "Init Tables": Value Change {
            n306 = event-data() -> ()  [unwired: 1 in, 6 out]
            n307 = call "System Parameters - FGV.vi"("Actions"=FGV_Actions."Get", "Error In"=w870) -> ("Error Out"=w869:errorcluster, "System Parameters [Out]"=w868:T33)  [unwired: 8 in]
            n308 = Unbundle By Name(w868) -> ("Table Stages"=w855:T23)
            n309 = call "XYZ Table Stage Module.vi"("Set/Get"=Set_Get_Controls."Set", "Action"=Motion_Translation_Module_Control2."Init", "Error In"=w869, "Axis"=enum16{"X Axis", "Y Axis", "Z Axis"}."X Axis", "Table Stages"=w855) -> ("Error Out"=w890:errorcluster)  [unwired: 5 in, 1 out]
            n310 = call "XYZ Table Stage Module.vi"("Set/Get"=Set_Get_Controls."Set", "Action"=Motion_Translation_Module_Control2."Init", "Error In"=w890, "Axis"=enum16{"X Axis", "Y Axis", "Z Axis"}."Y Axis", "Table Stages"=w855) -> ("Error Out"=w891:errorcluster)  [unwired: 5 in, 1 out]
            n311 = call "XYZ Table Stage Module.vi"("Set/Get"=Set_Get_Controls."Set", "Action"=Motion_Translation_Module_Control2."Init", "Error In"=w891, "Axis"=enum16{"X Axis", "Y Axis", "Z Axis"}."Z Axis", "Table Stages"=w855) -> ("Error Out"=w857:errorcluster)  [unwired: 5 in, 1 out]
            n312 = Unbundle By Name(w855) -> ("Attenuator"=w854:T24)
            n313 = call "refnum variable.vi"("action"=refnum_control."Get", "error in (no error)"=w857) -> ("error out"=w860:errorcluster, "reference in 2"=w859:refnum<k24>)  [unwired: 8 in]
            n314 = call "Cage controller.vi"("Set/Get"=Set_Get_Controls."Set", "error in (no error)"=w860, "Cluster In"=w854, "Action"=Motion_Translation_Module_Control2."Init", "reference in"=w859) -> ("error out"=w856:errorcluster)  [unwired: 4 in, 2 out]
            n315 = call "XYZ Table Stage Module.vi"("Set/Get"=Set_Get_Controls."Set", "Action"=Motion_Translation_Module_Control2."Velocity/Accel", "Error In"=w856, "Axis"=enum16{"X Axis", "Y Axis", "Z Axis"}."X Axis", "Table Stages"=w855) -> ("Error Out"=w892:errorcluster)  [unwired: 5 in, 1 out]
            n316 = call "XYZ Table Stage Module.vi"("Set/Get"=Set_Get_Controls."Set", "Action"=Motion_Translation_Module_Control2."Velocity/Accel", "Error In"=w892, "Axis"=enum16{"X Axis", "Y Axis", "Z Axis"}."Y Axis", "Table Stages"=w855) -> ("Error Out"=w893:errorcluster)  [unwired: 5 in, 1 out]
            n317 = call "XYZ Table Stage Module.vi"("Set/Get"=Set_Get_Controls."Set", "Action"=Motion_Translation_Module_Control2."Velocity/Accel", "Error In"=w893, "Axis"=enum16{"X Axis", "Y Axis", "Z Axis"}."Z Axis", "Table Stages"=w855) -> ("Error Out"=w864:errorcluster)  [unwired: 5 in, 1 out]
            n318 = call "Queue Manager.vi"("Queue Name"=QueueNames."Main GUI", "Action"=Queue_Manager_Actions."Enqueue", "Error In"=w864, "Message Packet Array"=T30[] [{"Message"="Wait for User Input", "Parameter"=variant}]) -> ("Error Out"=w863:errorcluster)  [unwired: 3 in, 4 out]
          }
          event Value Change {
            n319 = event-data() -> ("NewVal"=w896:bool)  [unwired: 1 in, 5 out]
            n320 = case shown="True" w896 {
              tunnel: w895 -> [w898 w909]
              tunnel: [w897 w907] -> w894
              frame False {
                n321 = call "Queue Manager.vi"("Queue Name"=QueueNames."Main GUI", "Action"=Queue_Manager_Actions."Enqueue", "Error In"=w898, "Message Packet Array"=T30[] [{"Message"="Wait for User Input", "Parameter"=variant}]) -> ("Error Out"=w897:errorcluster)  [unwired: 3 in, 4 out]
              }
              frame True {
                n322 = call "System Parameters - FGV.vi"("Actions"=FGV_Actions."Get", "Error In"=w909) -> ("Error Out"=w910:errorcluster, "System Parameters [Out]"=w908:T33)  [unwired: 8 in]
                n323 = call "Queue Manager.vi"("Queue Name"=QueueNames."Main GUI", "Action"=Queue_Manager_Actions."Enqueue", "Error In"=w910, "Message Packet Array"=T30[] [{"Message"="Wait for User Input", "Parameter"=variant}]) -> ("Error Out"=w906:errorcluster)  [unwired: 3 in, 4 out]
                n324 = Unbundle By Name(w908) -> ("Table Stages"=w903:T23, "Table Stages.Y Stage.Position"=w902:dbl)
                n325 = call "Y stage safety.vi"("new position"=w902, "Error In"=w906, "Table Stages"=w903) -> ("Error Out"=w905:errorcluster, "crash?"=w904:bool)  [unwired: 7 in]
                n326 = case shown="False" w904 {
                  tunnel: w903 -> [_ w927]
                  tunnel: w905 -> [w915 w922]
                  tunnel: [w915 w921] -> w907
                  frame True {
                    n327 = Two Button Dialog(message="Warning: about to crash!!! Movement invalid" ("T button name (\"OK\")"), 1:"Abort" ("F button name (\"Cancel\")"), 2:"Abort" ("T button name (\"OK\")")) -> ()  [unwired: 1 out]
                  }
                  frame False {
                    n328 = call "XYZ Table Stage Module.vi"("Set/Get"=Set_Get_Controls."Set", "Action"=Motion_Translation_Module_Control2."Velocity/Accel", "Error In"=w922, "Axis"=enum16{"X Axis", "Y Axis", "Z Axis"}."Y Axis", "Table Stages"=w927) -> ("Error Out"=w923:errorcluster, "Table Stages [out]"=w924:T23)  [unwired: 5 in]
                    n329 = call "XYZ Table Stage Module.vi"("Set/Get"=Set_Get_Controls."Set", "Action"=Motion_Translation_Module_Control2."Position", "Error In"=w923, "Axis"=enum16{"X Axis", "Y Axis", "Z Axis"}."Y Axis", "Table Stages"=w924) -> ("Error Out"=w921:errorcluster)  [unwired: 5 in, 1 out]
                  }
                }
              }
            }
          }
          event Value Change {
            n330 = event-data() -> ("NewVal"=w932:bool)  [unwired: 1 in, 5 out]
            n331 = case shown="True" w932 {
              tunnel: w931 -> [w934 w945]
              tunnel: [w933 w943] -> w930
              frame False {
                n332 = call "Queue Manager.vi"("Queue Name"=QueueNames."Main GUI", "Action"=Queue_Manager_Actions."Enqueue", "Error In"=w934, "Message Packet Array"=T30[] [{"Message"="Wait for User Input", "Parameter"=variant}]) -> ("Error Out"=w933:errorcluster)  [unwired: 3 in, 4 out]
              }
              frame True {
                n333 = call "System Parameters - FGV.vi"("Actions"=FGV_Actions."Get", "Error In"=w945) -> ("Error Out"=w946:errorcluster, "System Parameters [Out]"=w944:T33)  [unwired: 8 in]
                n334 = call "Queue Manager.vi"("Queue Name"=QueueNames."Main GUI", "Action"=Queue_Manager_Actions."Enqueue", "Error In"=w946, "Message Packet Array"=T30[] [{"Message"="Wait for User Input", "Parameter"=variant}]) -> ("Error Out"=w942:errorcluster)  [unwired: 3 in, 4 out]
                n335 = Unbundle By Name(w944) -> ("Table Stages.Z Stage.Position"=w938:dbl, "Table Stages"=w940:T23)
                n336 = call "Z stage safety.vi"("new position"=w938, "Error In"=w942, "Table Stages"=w940) -> ("Error Out"=w941:errorcluster, "crash?"=w939:bool)  [unwired: 7 in]
                n337 = case shown="True" w939 {
                  tunnel: w940 -> [_ w963]
                  tunnel: w941 -> [w951 w958]
                  tunnel: [w951 w957] -> w943
                  frame True {
                    n338 = Two Button Dialog(message="Warning: about to crash!!! Movement invalid" ("T button name (\"OK\")"), 1:"Abort" ("F button name (\"Cancel\")"), 2:"Abort" ("T button name (\"OK\")")) -> ()  [unwired: 1 out]
                  }
                  frame False {
                    n339 = call "XYZ Table Stage Module.vi"("Set/Get"=Set_Get_Controls."Set", "Action"=Motion_Translation_Module_Control2."Velocity/Accel", "Error In"=w958, "Axis"=enum16{"X Axis", "Y Axis", "Z Axis"}."Z Axis", "Table Stages"=w963) -> ("Error Out"=w959:errorcluster, "Table Stages [out]"=w960:T23)  [unwired: 5 in]
                    n340 = call "XYZ Table Stage Module.vi"("Set/Get"=Set_Get_Controls."Set", "Action"=Motion_Translation_Module_Control2."Position", "Error In"=w959, "Axis"=enum16{"X Axis", "Y Axis", "Z Axis"}."Z Axis", "Table Stages"=w960) -> ("Error Out"=w957:errorcluster)  [unwired: 5 in, 1 out]
                  }
                }
              }
            }
          }
          event "Quit": Value Change {
            (unwired) FALSE ("Status In")
            n341 = event-data() -> ()  [unwired: 1 in, 1 out]
            n342 = call "FGV - Acquisition Status.vi"("Actions"=FGV_Actions."Get", "Error In"=w971) -> ("Error Out"=w970:errorcluster, "Scan Type [Out]"=w968:T6, "mem loc out"=w966:i32)  [unwired: 6 in, 1 out]
            n343 = call "FGV - Acquisition Status.vi"("mem loc"=w966, "Actions"=FGV_Actions."Set", "Error In"=w970, "Quit status"=TRUE, "Scan Type [In]"=w968) -> ("Error Out"=w969:errorcluster)  [unwired: 3 in, 3 out]
            n344 = call "Queue Manager.vi"("Action"=Queue_Manager_Actions."Flush All Queues", "Error In"=w969) -> ("Error Out"=w974:errorcluster)  [unwired: 5 in, 4 out]
            n345 = call "Status Queue.vi"("Action"=Queue_Manager_Actions."Enqueue", "Error In"=w974, "Status Message [In]"="Exiting Software...See you later Stephan") -> ("Error Out"=w978:errorcluster)  [unwired: 7 in, 1 out]
            n346 = disable-structure shown="Enabled" {
              disable-tunnel: w978 -> [w985 w986]
              disable-tunnel: [w984 w986] -> w977
              frame Disabled {
                n347 = call "Set Main GUI for Different Acquire States.vi"("Error In"=w985, "Scan Type [Out]"=ScanType."Single Frame") -> ("Error Out"=w984:errorcluster)  [unwired: 9 in]
              }
              frame Enabled {
              }
            }
            n348 = call "Queue Manager.vi"("Action"=Queue_Manager_Actions."Enqueue All", "Error In"=w977, "Message Packet Array"=T30[] [{"Message"="Exit", "Parameter"=variant}] ("Message Packet [In]")) -> ("Error Out"=w982:errorcluster)  [unwired: 4 in, 4 out]
          }
          event Value Change {
            n349 = event-data() -> ("NewVal"=w987:bool)  [unwired: 1 in, 5 out]
            n350 = call "Pause.vi"("action"=Pause_action."set", "error in"=w993, "Pause!"=w987) -> ("error out"=w989:errorcluster)  [unwired: 7 in, 1 out]
            n351 = call "Queue Manager.vi"("Queue Name"=QueueNames."Main GUI", "Action"=Queue_Manager_Actions."Enqueue", "Error In"=w989, "Message Packet Array"=T30[] [{"Message"="Wait for User Input", "Parameter"=variant}]) -> ("Error Out"=w988:errorcluster)  [unwired: 3 in, 4 out]
          }
          event "AIP": Value Change {
            w1003 = 2 items=["No Event"=0, "Click Event"=1, "Draw Event"=2, "Size Event"=4, "Scroll Event"=5, "Double Click Event"=8]
            n352 = event-data() -> ("CtlRef"=w995:refnum<vi>)  [unwired: 1 in, 5 out]
            n353 = Build Array(w1003) -> (w1004:i32[])
            n354 = invoke class="ImageControl" method="Get Last Event"(reference=w995, error in=w1002, "Which Events"=w1004) -> (error out=w1001:errorcluster)  [unwired: 5 in, 7 out]
            n355 = Build Array(T30 {"Message"="Wait for User Input", "Parameter"=variant} ("Message Packet [In]")) -> (w996:T30[])
            n356 = call "Queue Manager.vi"("Queue Name"=QueueNames."Main GUI", "Action"=Queue_Manager_Actions."Enqueue", "Error In"=w1001, "Message Packet Array"=w996) -> ("Error Out"=w1000:errorcluster)  [unwired: 3 in, 4 out]
          }
          event Value Change {
            n357 = event-data() -> ("NewVal"=w1009:T44)  [unwired: 1 in]
            n358 = Add(x=w1009, y=5) -> (x+y=w1022:i32)
            n359 = call "System Parameters - FGV.vi"("Actions"=FGV_Actions."Get", "Error In"=w1013) -> ("Error Out"=w1012:errorcluster, "System Parameters [Out]"=w1010:T33)  [unwired: 8 in]
            n360 = Power Of 2(x=w1022) -> (2^x=w1021:dbl)
            n361 = local read "Imaging Parameter"() -> (w1008:T4)
            n362 = To Unsigned Word Integer(number=w1021) -> (unsigned 16bit integer=w1006:u16)
            n363 = Bundle By Name(cluster=w1010, "Imaging Parameter.XY Image Size"=w1009) -> (w1005:T33)
            n364 = Bundle By Name(cluster=w1008, "Custom Size.X"=w1006, "Custom Size.Y"=w1006) -> (w1007:T4)
            n365 = local write "Imaging Parameter"(w1007) -> ()
            n366 = call "System Parameters - FGV.vi"("Actions"=FGV_Actions."Set", "Error In"=w1012, "System Parameters [In]"=w1005) -> ("Error Out"=w1011:errorcluster)  [unwired: 7 in, 1 out]
            n367 = Build Array(T30 {"Message"="Wait for User Input", "Parameter"=variant} ("Message Packet [In]")) -> (w1017:T30[])
            n368 = call "Queue Manager.vi"("Queue Name"=QueueNames."Main GUI", "Action"=Queue_Manager_Actions."Enqueue", "Error In"=w1011, "Message Packet Array"=w1017) -> ("Error Out"=w1016:errorcluster)  [unwired: 3 in, 4 out]
          }
          event Value Change {
            n369 = event-data() -> ()  [unwired: 1 in, 6 out]
            n370 = call "FGV - Acquisition Status.vi"("Actions"=FGV_Actions."Get") -> ("mem loc out"=w1024:i32)  [unwired: 7 in, 3 out]
            n371 = call "FGV - Acquisition Status.vi"("mem loc"=w1024, "Actions"=FGV_Actions."Set", "Quit status"=FALSE, "Scan Type [In]"="Scan Type") -> ()  [unwired: 4 in, 4 out]
            n372 = call "Queue Manager.vi"("Queue Name"=QueueNames."Main GUI", "Action"=Queue_Manager_Actions."Enqueue", "Error In"=w1033, "Message Packet Array"=T30[] [{"Message"="Set Front Panel", "Parameter"=variant}, {"Message"="Wait for User Input", "Parameter"=variant}]) -> ("Error Out"=w1029:errorcluster)  [unwired: 3 in, 4 out]
          }
          event "Acquire": Value Change {
            n373 = event-data() -> ()  [unwired: 1 in, 6 out]
            n374 = call "Queue Manager.vi"("Queue Name"=QueueNames."Main GUI", "Action"=Queue_Manager_Actions."Enqueue", "Error In"=w1046, "Message Packet Array"=T30[] [{"Message"="Wait for User Input", "Parameter"=variant}]) -> ("Error Out"=w1034:errorcluster)  [unwired: 3 in, 4 out]
            n375 = call "FGV - Acquisition Status.vi"("Actions"=FGV_Actions."Get", "Error In"=w1034) -> ("Error Out"=w1038:errorcluster, "Scan Type [Out]"=w1039:T6, "mem loc out"=w1036:i32)  [unwired: 6 in, 1 out]
            n376 = call "FGV - Acquisition Status.vi"("mem loc"=w1036, "Actions"=FGV_Actions."Set", "Error In"=w1038, "Quit status"=FALSE, "Scan Type [In]"=w1039) -> ()  [unwired: 3 in, 4 out]
            n377 = case "Start Acquisition?" shown="False" FALSE {
              tunnel: w1034 -> [w1047 w1055]
              tunnel: [w1048 w1055] -> w1045
              frame False {
                # "Starts Acquisition if Current Acquisition Status is \"Off\""
                n378 = call "Queue Manager.vi"("Queue Name"=QueueNames."Main Scan Processor", "Action"=Queue_Manager_Actions."Enqueue", "Error In"=w1047, "Message Packet Array"=T30[] [{"Message"="Acquire", "Parameter"=variant}] ("Message Packet [In]")) -> ("Error Out"=w1049:errorcluster)  [unwired: 3 in, 4 out]
                n379 = call "Status Queue.vi"("Action"=Queue_Manager_Actions."Enqueue", "Error In"=w1049, "Status Message [In]"="Scanning...") -> ("Error Out"=w1048:errorcluster)  [unwired: 7 in, 1 out]
              }
              frame True {
                # "Stops Acquisition if Current Status is On"
              }
            }
          }
        }
      }
      frame "Exit" {
        n380 = call "System Parameters - FGV.vi"("Actions"=FGV_Actions."Get", "Error In"=w1064) -> ("Error Out"=w1063:errorcluster, "System Parameters [Out]"=w1056:T33)  [unwired: 8 in]
        n381 = call "Write Config to File.vi"("error in (no error)"=w1063, "System Parameters"=w1056) -> ("error out"=w1059:errorcluster)  [unwired: 9 in]
        n382 = call "Save Data Queue.vi"("Action"=Queue_Manager_Actions."Release Queue", "error in (no error)"=w1059) -> ("error out"=w1058:errorcluster)  [unwired: 6 in, 3 out]
        n383 = Unbundle By Name(w1056) -> ("Table Stages"=w1061:T23)
        n384 = disable-structure shown="Enabled" {
          disable-tunnel: w1061 -> [w1072 _]
          disable-tunnel: w1058 -> [w1069 w1084]
          disable-tunnel: [w1066 w1084] -> w1057
          frame Disabled {
            n385 = call "XYZ Table Stage Module.vi"("Set/Get"=Set_Get_Controls."Set", "Action"=Motion_Translation_Module_Control2."Uninit", "Error In"=w1069, "Axis"=enum16{"X Axis", "Y Axis", "Z Axis"}."Z Axis", "Table Stages"=w1072) -> ("Error Out"=w1077:errorcluster, "Table Stages [out]"=w1071:T23)  [unwired: 5 in]
            n386 = call "XYZ Table Stage Module.vi"("Set/Get"=Set_Get_Controls."Set", "Action"=Motion_Translation_Module_Control2."Uninit", "Error In"=w1077, "Axis"=enum16{"X Axis", "Y Axis", "Z Axis"}."Y Axis", "Table Stages"=w1071) -> ("Error Out"=w1076:errorcluster, "Table Stages [out]"=w1070:T23)  [unwired: 5 in]
            n387 = call "XYZ Table Stage Module.vi"("Set/Get"=Set_Get_Controls."Set", "Action"=Motion_Translation_Module_Control2."Uninit", "Error In"=w1076, "Axis"=enum16{"X Axis", "Y Axis", "Z Axis"}."X Axis", "Table Stages"=w1070) -> ("Error Out"=w1067:errorcluster)  [unwired: 5 in, 1 out]
            n388 = call "Cage controller.vi"("error in (no error)"=w1067, "Action"=Motion_Translation_Module_Control2."Uninit") -> ("error out"=w1066:errorcluster)  [unwired: 7 in, 2 out]
          }
          frame Enabled {
          }
        }
      }
      frame Default {
      }
    }
    n389 = call "Error Message Handler.vi"("Error In"=w589) -> ("Error Out"=w592:errorcluster, "T button?"=w591:bool)  [unwired: 9 in]
    n390 = case shown="False" w591 {
      tunnel: w592 -> [w601 w602]
      tunnel: [w601 w603] -> w590
      frame False {
      }
      frame True {
        n391 = call "Status Queue.vi"("Action"=Queue_Manager_Actions."Enqueue", "Error In"=w602, "Status Message [In]"="Exiting Software...") -> ("Error Out"=w607:errorcluster)  [unwired: 7 in, 1 out]
        n392 = call "Set Main GUI for Different Acquire States.vi"("Error In"=w607, "Scan Type [Out]"=ScanType."Single Frame") -> ("Error Out"=w606:errorcluster)  [unwired: 9 in]
        n393 = call "Queue Manager.vi"("Action"=Queue_Manager_Actions."Enqueue All", "Error In"=w606, "Message Packet Array"=T30[] [{"Message"="Exit", "Parameter"=variant}] ("Message Packet [In]")) -> ("Error Out"=w603:errorcluster)  [unwired: 4 in, 4 out]
      }
    }
  }
  n394 = call "Queue Manager.vi"("Queue Name"=QueueNames."Main Display", "Action"=Queue_Manager_Actions."Release Queue", "Error In"=w14) -> ()  [unwired: 4 in, 5 out]
  n395 = call "Queue Manager.vi"("Queue Name"=QueueNames."Main Processing", "Action"=Queue_Manager_Actions."Release Queue", "Error In"=w9) -> ()  [unwired: 4 in, 5 out]
  n396 = call "File log.vi"("action"=T27."Close file", "error in"=w4) -> ("error out"=w3:errorcluster)  [unwired: 9 in]
  n397 = call "Queue Manager.vi"("Queue Name"=QueueNames."Main Scan Processor", "Action"=Queue_Manager_Actions."Release Queue", "Error In"=w16) -> ()  [unwired: 4 in, 5 out]
  n398 = call "Queue Manager.vi"("Queue Name"=QueueNames."Main Saving", "Action"=Queue_Manager_Actions."Release Queue", "Error In"=w3) -> ()  [unwired: 4 in, 5 out]
  n399 = call "Queue Manager.vi"("Queue Name"=QueueNames."Main GUI", "Action"=Queue_Manager_Actions."Release Queue", "Error In"=w21) -> ()  [unwired: 4 in, 5 out]
  "wanring" <- "if using GPU FFT, FOV size should be smaller than 2000x2000(including A-line and B-line averaging), due to RAM limit" ("String")
